vi "VentTrainer.vi"() -> ()   [LabVIEW 2019]
uses:
  <vilib>/Utility/miscctls.llb/LVForegroundBackgroundColorsTypeDef.ctl
  <vilib>/Utility/miscctls.llb/LVTextColorsTypeDef.ctl
  <vilib>/Platform/TimedLoop/XDataNode/timing_clust.ctl
  <vilib>/Platform/TimedLoop/XDataNode/nitl_modes.ctl
  <vilib>/Platform/TimedLoop/XDataNode/wakeup.ctl
  <vilib>/imath/engines/lvmath/Plug In/_Char/NIMS_CH_character datatype.ctl
  <vilib>/numeric/Random Number (Range) U64.vi
  <vilib>/numeric/sub_Random U32.vi
  <vilib>/imath/engines/lvmath2/RunTimeEngine/Managers/WorkSpace/UID Generator.vi
  <vilib>/imath/engines/lvmath2/RunTimeEngine/BuiltInFunctions/le/NIMS_le_no_size_check.vi
  <instcachedir>/0/NIMS_le_no_size_check_D856ED23C6134ED1894787F1ECBE09FB.lvgen/NIMS_le_no_size_check_D856ED23C6134ED1894787F1ECBE09FB_000.vi
  <vilib>/imath/engines/lvmath2/RunTimeEngine/BuiltInFunctions/gt/NIMS_gt_no_size_check.vi
  <instcachedir>/0/NIMS_gt_no_size_check_38A9727757664B91B08F4CCA058B820F.lvgen/NIMS_gt_no_size_check_38A9727757664B91B08F4CCA058B820F_000.vi
  <vilib>/imath/engines/lvmath2/RunTimeEngine/RunTimeType/NIMS_RunTimeType_From StrictType (excl LVString).vi
  <instcachedir>/0/NIMS_RunTimeType_From StrictType (excl LVString)_D8AFBA86A94845AAA577C895450664BD.lvgen/NIMS_RunTimeType_From StrictType (excl LVString)_D8AFBA86A94845AAA577C895450664BD_000.vi
  <vilib>/imath/engines/lvmath2/RunTimeEngine/LocalVariableDefStatement/MC_LocalVariableDefStatement_Display.vi
  <vilib>/imath/engines/lvmath2/RunTimeEngine/Managers/SymbolTable/Clear UID.vi
  <vilib>/imath/engines/lvmath2/RunTimeEngine/NodeEndStatement/NIMS_NodeEndStatement_Output.vi
  <instcachedir>/0/NIMS_NodeEndStatement_Output_53EC0D466D134D7ABD903AC30B43404B.lvgen/NIMS_NodeEndStatement_Output_53EC0D466D134D7ABD903AC30B43404B_001.vi
  <vilib>/imath/engines/lvmath2/RunTimeEngine/ErrorHandling/NIMS_Finalize Error.vi
  <vilib>/imath/engines/lvmath2/RunTimeEngine/BuiltInFunctions/lt/NIMS_lt_no_size_check.vi
  <instcachedir>/0/NIMS_lt_no_size_check_D875779DF14246DBB85DAA0AEACCEBA5.lvgen/NIMS_lt_no_size_check_D875779DF14246DBB85DAA0AEACCEBA5_000.vi
  <vilib>/imath/engines/lvmath/Plug In/_Char/NIMS_CH_Character RV to String.vi
  <instcachedir>/0/NIMS_NodeEndStatement_Output_53EC0D466D134D7ABD903AC30B43404B.lvgen/NIMS_NodeEndStatement_Output_53EC0D466D134D7ABD903AC30B43404B_008.vi
  <instcachedir>/0/NIMS_NodeEndStatement_Output_53EC0D466D134D7ABD903AC30B43404B.lvgen/NIMS_NodeEndStatement_Output_53EC0D466D134D7ABD903AC30B43404B_010.vi
  <vilib>/imath/engines/lvmath2/RunTimeEngine/BuiltInFunctions/ge/NIMS_ge_no_size_check.vi
  <instcachedir>/0/NIMS_ge_no_size_check_103862EFDADA4303A5E7B19FE76B9AA5.lvgen/NIMS_ge_no_size_check_103862EFDADA4303A5E7B19FE76B9AA5_000.vi
  <vilib>/imath/engines/lvmath2/RunTimeEngine/BuiltInFunctions/rem/NIMS_rem_no checks.vi
  <instcachedir>/0/NIMS_rem_no checks_044AAE96F86F43668F02B1B11ED2BED0.lvgen/NIMS_rem_no checks_044AAE96F86F43668F02B1B11ED2BED0_000.vi
  <vilib>/imath/engines/lvmath2/RunTimeSupport/NIMS_Error if Not Equal.vi
  <instcachedir>/0/NIMS_Error if Not Equal_D50A0F08CBFC40E0B64682CCD852CBC7.lvgen/NIMS_Error if Not Equal_D50A0F08CBFC40E0B64682CCD852CBC7_000.vi
  <vilib>/imath/engines/lvmath2/RunTimeEngine/IndexReplace/NIMS V(S)=S.vi
  <instcachedir>/0/NIMS V(S)=S_BD5C8CB81B6E4D99B8C0034EA1BEE55D.lvgen/NIMS V(S)=S_BD5C8CB81B6E4D99B8C0034EA1BEE55D_000.vi
  <vilib>/imath/engines/lvmath2/RunTimeEngine/ErrorHandling/NIMS_Create Error From Enums.vi
  <vilib>/imath/engines/lvmath2/RunTimeEngine/RangeToken/NIMS_Range_R2 - Integer.vi
  <instcachedir>/0/NIMS_Range_R2 - Integer_8A7AF97FD8504F909FC0FDE0F1D1FB54.lvgen/NIMS_Range_R2 - Integer_8A7AF97FD8504F909FC0FDE0F1D1FB54_000.vi
  <vilib>/imath/engines/lvmath2/RunTimeEngine/CommandStatement/MC_CommandStatement_break.vi
  <vilib>/imath/engines/lvmath2/RunTimeEngine/IndexRead/NIMS V(S).vi
  <instcachedir>/0/NIMS V(S)_0488751826AF41519A22953C041130DC.lvgen/NIMS V(S)_0488751826AF41519A22953C041130DC_000.vi
  <vilib>/imathl/engines/lvmath/Functions/Error Handling/Create Error.vi
  <vilib>/imath/engines/lvmath2/RunTimeEngine/VariableToken/NIMS_VariableToken_CondDefined.vi
  <instcachedir>/0/NIMS_VariableToken_CondDefined_30C3C94EAC01413DA882E848DEC89944.lvgen/NIMS_VariableToken_CondDefined_30C3C94EAC01413DA882E848DEC89944_003.vi
  <vilib>/imath/engines/lvmath/Functions/Error Handling/MergeErrorsWrapper.vi
  <instcachedir>/0/NIMS_NodeEndStatement_Output_53EC0D466D134D7ABD903AC30B43404B.lvgen/NIMS_NodeEndStatement_Output_53EC0D466D134D7ABD903AC30B43404B_005.vi
  <instcachedir>/0/NIMS_NodeEndStatement_Output_53EC0D466D134D7ABD903AC30B43404B.lvgen/NIMS_NodeEndStatement_Output_53EC0D466D134D7ABD903AC30B43404B_011.vi
  <instcachedir>/0/NIMS V(S)=S_BD5C8CB81B6E4D99B8C0034EA1BEE55D.lvgen/NIMS V(S)=S_BD5C8CB81B6E4D99B8C0034EA1BEE55D_003.vi
  <vilib>/imath/engines/lvmath2/RunTimeEngine/RangeToken/NIMS_Range_R2 - Float.vi
  <instcachedir>/0/NIMS_Range_R2 - Float_E92E97654E134110B10F16A3994F6405.lvgen/NIMS_Range_R2 - Float_E92E97654E134110B10F16A3994F6405_000.vi
  <vilib>/imath/engines/lvmath2/RunTimeEngine/BuiltInFunctions/eq/NIMS_eq_no_size_check.vi
  <instcachedir>/0/NIMS_eq_no_size_check_3C30971638434A0885768DE8C65273EC.lvgen/NIMS_eq_no_size_check_3C30971638434A0885768DE8C65273EC_000.vi
  <instcachedir>/0/NIMS_NodeEndStatement_Output_53EC0D466D134D7ABD903AC30B43404B.lvgen/NIMS_NodeEndStatement_Output_53EC0D466D134D7ABD903AC30B43404B_012.vi
  <instcachedir>/0/NIMS_NodeEndStatement_Output_53EC0D466D134D7ABD903AC30B43404B.lvgen/NIMS_NodeEndStatement_Output_53EC0D466D134D7ABD903AC30B43404B_018.vi
  <vilib>/platform/TimedLoop/XDataNode/XDataNode.xnode
  <vilib>/Platform/TimedLoop/XDataNode/XDNodeRunTimeDep.lvlib
  <vilib>/imath/engines/lvmath2/RunTimeEngine/Managers/SymbolTable/NIMS_WorkSpace.lvlib
panel:
  out "flagTime1 2":bool
  out "countCycle":dbl
  out "flagTime3":bool
  out "flagTime2":bool
  out "flagTime1":bool
  out "startSimu":bool
  out "indexRef":dbl=1.0
  out "scenTrigger":bool
  out "currentTime":u32=43420372
  out "StringPressure":string="Paw: NaN [cmH2O]\r\nTempo: 0.50 [s]"
  out "StringFlow":string="Fluxo: NaN [l/min]\r\nTempo: 0.50 [s]"
  out "StringVolume":string="Volume: NaN [ml]\r\nTempo: 0.50 [s]"
  out "sizeArray":i32=678
  in  "background":enum32{"Page 1"}(tab)
  in  "info":bool
  out "Bat. %":u8(slide)=100 scale=0.0..100.0
  in  "confTab":enum32{"CONFIGURAÇÕES"}(tab)
  in  "Cenários":u16(ring) items=["Livre", "Cenário 1", "Cenário 2", "Cenário 3", "Cenário 4", "Cenário 5"]
  in  "runBtn":bool
  in  "pacienteTab":T1(tab)
  out "Peso Ideal (kg)":dbl=75.116 format="%_4g"
  in  "Peso (kg)":u16=70 min=1 max=500 step=1
  in  "Altura (m)":dbl=1.8 min=0.1 max=2.8 step=0.1 format="%_2f"
  in  "Idade (anos)":u8=42 min=1 max=120 step=1
  in  "Sexo":u16(ring) items=["Masculino", "Feminino"]
  in  "enbPmus":bool
  in  "enbPalv":bool
  in  "Tempo de Simulação [s]":u8(slide)=10 min=5 max=30 step=5 scale=5.0..30.0
  in  "Rva [cmH2O/l/s]":u8(slide)=10 min=5 max=50 step=2 scale=5.0..50.0
  in  "Cst [ml/cmH2O]":u8(slide)=20 min=5 max=60 step=2 scale=5.0..60.0
  in  "Pausa Inspiratória [s]":dbl(slide) min=0.0 max=5.0 step=0.1 scale=0.0..5.0
  in  "Pmus [cmH2O]":dbl(slide)=2.0999999999999996 min=0.0 max=10.0 step=0.1 scale=0.0..10.0
  in  "stimBtn":bool
  out "spo2":string="SpO2: 97"
  out "alarm_text":string="1  BATERIA fraca"
  in  "ventMode":enum32{"VCV", "PCV"}(tab)
  in  "vcv_blend_up":bool
  in  "vcv_blend_down":bool
  out "vcv_fio2":i16=100
  in  "sens_up":bool
  in  "sens_down":bool
  out "vcv_sens":dbl=-3.0 format="%_2g"
  in  "peep_up":bool
  in  "peep_down":bool
  out "vcv_peep":i16=5
  in  "freq_up":bool
  in  "freq_down":bool
  out "vcv_freq":i16=20
  in  "flow_up":bool
  in  "flow_down":bool
  out "vcv_flow":i16=24
  in  "volume_up":bool
  in  "volume_down":bool
  out "vcv_volume":i16=450
  in  "pc_up":bool
  in  "pc_down":bool
  out "pcv_pc":i16=10
  in  "tinsp_up":bool
  in  "tinsp_down":bool
  out "pcv_tinsp":dbl=1.0 format="%_2g"
  in  "freq_up":bool
  in  "freq_down":bool
  out "pcv_freq":i16=15
  in  "rise_up":bool
  in  "rise_down":bool
  out "pcv_rise":dbl=0.25 format="%.2f"
  in  "peep_up":bool
  in  "peep_down":bool
  out "pcv_peep":i16=5
  in  "sens_up":bool
  in  "sens_down":bool
  out "pcv_sens":dbl=-3.0 format="%_2g"
  in  "blend_up":bool
  in  "blend_down":bool
  out "pcv_blend":i8=100
  in  "monTab":enum32{"MON. 1", "MON. 2"}(tab)
  in  "lowPeak":i16=10 min=0 max=2000 step=1
  in  "highPeak":i16=35 min=0 max=2000 step=1
  out "pPeak":i16
  out "vti":i16
  in  "highVti":i16=400 min=0 max=2000 step=1
  in  "lowVti":i16=200 min=0 max=2000 step=1
  out "ve":dbl format="%.1f"
  in  "highVe":dbl=10.0 min=0.0 max=20.0 step=0.1 format="%_2g"
  in  "lowVe":dbl=2.0 min=0.0 max=20.0 step=0.1 format="%_2f"
  in  "lowPeep":i16=2 min=0 max=2000 step=1
  in  "highPeep":i16=8 min=0 max=2000 step=1
  out "PEEP":dbl format="%_2g"
  in  "lowVte":i16=200 min=0 max=2000 step=1
  in  "highVte":i16=400 min=0 max=2000 step=1
  out "vte":i16
  in  "lowFio2":i16=60 min=21 max=99 step=1
  in  "highFio2":i16=80 min=21 max=100 step=1
  out "Fio2":i16
  out "IE":string="1:0.0"
  out "tInsp":dbl format="%_3g"
  in  "lowFreq":i16=10 min=0 max=2000 step=1
  in  "highFreq":i16=30 min=0 max=2000 step=1
  out "fTotal":i16
  out "pPlateau":dbl
  out "drivingP":dbl
  in  "lowFlow":i16=2 min=0 max=2000 step=1
  in  "highFlow":i16=30 min=0 max=2000 step=1
  out "pFlow":i16
  in  "graphsTab":enum32{"CURVAS", "LOOPs"}(tab)
  out "graph3":cluster{dbl[], dbl[]}[](graph)=[{array[678 elements], array[679 elements]}, {array[678 elements], array[703 elements]}, {array[678 elements], [nan, nan, nan, nan, nan, nan, nan, nan, nan, nan, nan, nan, nan, nan, nan, nan, nan, nan, nan, nan, nan, nan, nan, nan, nan, nan, nan, nan, nan, nan, nan, nan, nan, nan, nan, nan, nan, nan, nan, nan, nan, nan, nan, nan, nan, nan, nan, nan, nan, nan, nan, nan, nan, nan, nan, nan, nan, nan, nan, nan, nan, nan, nan, nan, nan, nan, nan, nan, nan, nan, nan, nan, nan, nan, nan, nan, nan, nan, nan, nan, nan, nan, nan, nan, nan, nan, nan, nan, nan, nan, nan, nan, nan, nan, nan, nan, nan, nan, nan, nan, nan, nan, nan, nan, nan, nan, nan, nan, nan, nan, nan, nan, nan, nan, nan, nan, nan, nan, nan, nan, nan, nan, nan, nan, nan, nan, nan, nan, nan, nan, nan, nan, nan, nan, nan, nan, nan, nan, nan, nan, nan, nan, nan, nan, nan, nan, nan, nan, nan, nan, nan, nan, nan, nan, nan, nan, nan, nan, nan, nan, nan, nan, nan, nan, nan, nan, nan, nan, nan, nan, nan, nan, nan, nan, nan, nan, nan, nan, nan, nan, nan, nan, nan, nan, nan, nan, nan, nan, nan, nan, nan, nan, nan, nan, nan, nan, nan, nan, nan, nan, nan, nan, nan, nan, nan, nan, nan, nan, nan, nan, nan, nan, nan, nan, nan, nan, nan, nan, nan, nan, nan, nan, nan, nan, nan, nan, nan, nan, nan, nan, nan, nan, nan, nan, nan, nan, nan, nan, nan, nan, nan, nan, nan, nan, nan, nan, nan, nan, nan, nan, nan, nan, nan, nan, nan, nan, nan, nan, nan, nan, nan, nan, nan, nan, nan, nan, nan, nan, nan, nan, nan, nan, nan, nan, nan, nan, nan, nan, nan, nan, nan, nan, nan, nan, nan, nan, nan, nan, nan, nan, nan, nan, nan, nan, nan, nan, nan, nan, nan, nan, nan, nan, nan, nan, nan, nan, nan, nan, nan, nan, nan, nan, nan, nan, nan, nan, nan, nan, nan, nan, nan, nan, nan, nan, nan, nan, nan, nan, nan, nan, nan, nan, nan, nan, nan, nan, nan, nan, nan, nan, nan, nan, nan, nan, nan, nan, nan, nan, nan, nan, nan, nan, nan, nan, nan, nan, nan, nan, nan, nan, nan, nan, nan, nan, nan, nan, nan, nan, nan, nan, nan, nan, nan, nan, nan, nan, nan, nan, nan, nan, nan, nan, nan, nan, nan, nan, nan, nan, nan, nan, nan, nan, nan, nan, nan, nan, nan, nan, nan, nan, nan, nan, nan, nan, nan, nan, nan, nan, nan, nan, nan, nan, nan, nan, nan, nan, nan, nan, nan, nan, nan, nan, nan, nan, nan, nan, nan, nan, nan, nan, nan, nan, nan, nan, nan, nan, nan, nan, nan, nan, nan, nan, nan, nan, nan, nan, nan, nan, nan, nan, nan, nan, nan, nan, nan, nan, nan, nan, nan, nan, nan, nan, nan, nan, nan, nan, nan, nan, nan, nan, nan, nan, nan, nan, nan, nan, nan, nan, nan, nan, nan, nan, nan, nan, nan, nan, nan, nan, nan, nan, nan, nan, nan, nan, nan, nan, nan, nan, nan, nan, nan, nan, nan, nan, nan, nan, nan, nan, nan, nan, nan, nan, nan, nan, nan, nan, nan, nan, nan, nan, nan, nan, nan, nan, nan, nan, nan, nan, nan, nan, nan, nan, nan, nan, nan, nan, nan, nan, nan, nan, nan, nan, nan, nan, nan, nan, nan, nan, nan, nan, nan, nan, nan, nan, nan, nan, nan, nan, nan, nan, nan, nan, nan, nan, nan, nan, nan, nan, nan, nan, nan, nan, nan, nan, nan, nan, nan, nan, nan, nan, nan, nan, nan, nan, nan, nan, nan, nan, nan, nan, nan, nan, nan, nan, nan, nan, nan, nan, nan, nan, nan, nan, nan, nan, nan, nan, nan, nan, nan, nan, nan, nan, nan, nan, nan, nan, nan, nan, nan, nan, nan, nan, nan, nan, nan, nan, nan, nan, nan, nan, nan, nan, nan, nan, nan, nan, nan, nan, nan, nan, nan, nan, nan, nan, nan, nan, nan, nan, nan, nan, nan, nan, nan, nan, nan, nan, nan, nan, nan, nan, nan, nan, nan, nan, nan, nan, nan, nan, nan, nan, nan, nan, nan, nan, nan, nan, nan, nan, nan, nan, nan, nan, nan, nan, nan, nan, nan, nan, nan, nan, nan, nan, nan, nan, nan, nan, nan, nan, nan, nan, nan, nan, nan]}, {array[678 elements], [nan, nan, nan, nan, nan, nan, nan, nan, nan, nan, nan, nan, nan, nan, nan, nan, nan, nan, nan, nan, nan, nan, nan, nan, nan, nan, nan, nan, nan, nan, nan, nan, nan, nan, nan, nan, nan, nan, nan, nan, nan, nan, nan, nan, nan, nan, nan, nan, nan, nan, nan, nan, nan, nan, nan, nan, nan, nan, nan, nan, nan, nan, nan, nan, nan, nan, nan, nan, nan, nan, nan, nan, nan, nan, nan, nan, nan, nan, nan, nan, nan, nan, nan, nan, nan, nan, nan, nan, nan, nan, nan, nan, nan, nan, nan, nan, nan, nan, nan, nan, nan, nan, nan, nan, nan, nan, nan, nan, nan, nan, nan, nan, nan, nan, nan, nan, nan, nan, nan, nan, nan, nan, nan, nan, nan, nan, nan, nan, nan, nan, nan, nan, nan, nan, nan, nan, nan, nan, nan, nan, nan, nan, nan, nan, nan, nan, nan, nan, nan, nan, nan, nan, nan, nan, nan, nan, nan, nan, nan, nan, nan, nan, nan, nan, nan, nan, nan, nan, nan, nan, nan, nan, nan, nan, nan, nan, nan, nan, nan, nan, nan, nan, nan, nan, nan, nan, nan, nan, nan, nan, nan, nan, nan, nan, nan, nan, nan, nan, nan, nan, nan, nan, nan, nan, nan, nan, nan, nan, nan, nan, nan, nan, nan, nan, nan, nan, nan, nan, nan, nan, nan, nan, nan, nan, nan, nan, nan, nan, nan, nan, nan, nan, nan, nan, nan, nan, nan, nan, nan, nan, nan, nan, nan, nan, nan, nan, nan, nan, nan, nan, nan, nan, nan, nan, nan, nan, nan, nan, nan, nan, nan, nan, nan, nan, nan, nan, nan, nan, nan, nan, nan, nan, nan, nan, nan, nan, nan, nan, nan, nan, nan, nan, nan, nan, nan, nan, nan, nan, nan, nan, nan, nan, nan, nan, nan, nan, nan, nan, nan, nan, nan, nan, nan, nan, nan, nan, nan, nan, nan, nan, nan, nan, nan, nan, nan, nan, nan, nan, nan, nan, nan, nan, nan, nan, nan, nan, nan, nan, nan, nan, nan, nan, nan, nan, nan, nan, nan, nan, nan, nan, nan, nan, nan, nan, nan, nan, nan, nan, nan, nan, nan, nan, nan, nan, nan, nan, nan, nan, nan, nan, nan, nan, nan, nan, nan, nan, nan, nan, nan, nan, nan, nan, nan, nan, nan, nan, nan, nan, nan, nan, nan, nan, nan, nan, nan, nan, nan, nan, nan, nan, nan, nan, nan, nan, nan, nan, nan, nan, nan, nan, nan, nan, nan, nan, nan, nan, nan, nan, nan, nan, nan, nan, nan, nan, nan, nan, nan, nan, nan, nan, nan, nan, nan, nan, nan, nan, nan, nan, nan, nan, nan, nan, nan, nan, nan, nan, nan, nan, nan, nan, nan, nan, nan, nan, nan, nan, nan, nan, nan, nan, nan, nan, nan, nan, nan, nan, nan, nan, nan, nan, nan, nan, nan, nan, nan, nan, nan, nan, nan, nan, nan, nan, nan, nan, nan, nan, nan, nan, nan, nan, nan, nan, nan, nan, nan, nan, nan, nan, nan, nan, nan, nan, nan, nan, nan, nan, nan, nan, nan, nan, nan, nan, nan, nan, nan, nan, nan, nan, nan, nan, nan, nan, nan, nan, nan, nan, nan, nan, nan, nan, nan, nan, nan, nan, nan, nan, nan, nan, nan, nan, nan, nan, nan, nan, nan, nan, nan, nan, nan, nan, nan, nan, nan, nan, nan, nan, nan, nan, nan, nan, nan, nan, nan, nan, nan, nan, nan, nan, nan, nan, nan, nan, nan, nan, nan, nan, nan, nan, nan, nan, nan, nan, nan, nan, nan, nan, nan, nan, nan, nan, nan, nan, nan, nan, nan, nan, nan, nan, nan, nan, nan, nan, nan, nan, nan, nan, nan, nan, nan, nan, nan, nan, nan, nan, nan, nan, nan, nan, nan, nan, nan, nan, nan, nan, nan, nan, nan, nan, nan, nan, nan, nan, nan, nan, nan, nan, nan, nan, nan, nan, nan, nan, nan, nan, nan, nan, nan, nan, nan, nan, nan, nan, nan, nan, nan, nan, nan, nan, nan, nan, nan, nan, nan, nan, nan, nan, nan, nan, nan, nan, nan, nan, nan, nan, nan, nan, nan, nan, nan, nan, nan, nan, nan, nan, nan, nan, nan, nan, nan, nan, nan, nan, nan, nan, nan, nan, nan, nan, nan, nan, nan, nan, nan, nan, nan, nan, nan, nan, nan, nan, nan, nan, nan]}]
  out "graph1":cluster{"vec_1":dbl[], "vec_2":dbl[]}[](graph)
  out "graph2":cluster{"vec_1":dbl[], "vec_3":dbl[]}[](graph)
  out "graph4":cluster{"vec_2":dbl[], "vec_4":dbl[]}(graph)
  out "graph5":cluster{"vec_2":dbl[], "vec_4":dbl[]}(graph)
  out "trigger":bool
  out "rstModel":bool
  out "flag1":bool
  out "timeRef1":dbl=0.5
  out "flag3":bool
  out "timeRef3":dbl=8.040000000000001
  out "flag2":bool
  out "timeRef2":dbl=6.96 format="%.2f"
  out "scaleTrigger":bool
  out "simuTime":u8=10
  out "minFlow":dbl=-98.76291251592673
  out "maxFlow":dbl=24.0
  out "initTime":u64=43388394
  out "graphPressure":dbl format="%.6f"
  # "FiO2"
  # "%"
  # "Sens"
  # "cmH2O"
  # "PEEP"
  # "cmH2O"
  # "Freq"
  # "rpm"
  # "Flow"
  # "L/min"
  # "Volume"
  # "ml"
  # "PC"
  # "cmH2O"
  # "T. Insp"
  # "s"
  # "Freq"
  # "rpm"
  # "Rise Time"
  # "s"
  # "PEEP"
  # "cmH2O"
  # "Sens"
  # "cmH2O"
  # "FiO2"
  # "%"
  # "P. Peak"
  # "cmH2O"
  # "VTI"
  # "ml"
  # "VE"
  # "L/min"
  # "PEEP"
  # "cmH2O"
  # "VTE"
  # "ml"
  # "FiO2"
  # "%"
  # "I:E"
  # "T. Insp"
  # "s"
  # "fTotal"
  # "rpm"
  # "P. Plateau"
  # "cmH2O"
  # "Driving P."
  # "cmH2O"
  # "Peak Flow"
  # "ml/min"
  # "Volume [ml]"
  # "Fluxo [l/min]"
  # "Pressão [cmH2O]"
  # "Tempo [s]"
  # "Volume [ml]"
  # "Pressão [cmH2O]"
  # "Fluxo [L/min]"
  # "Volume [ml]"
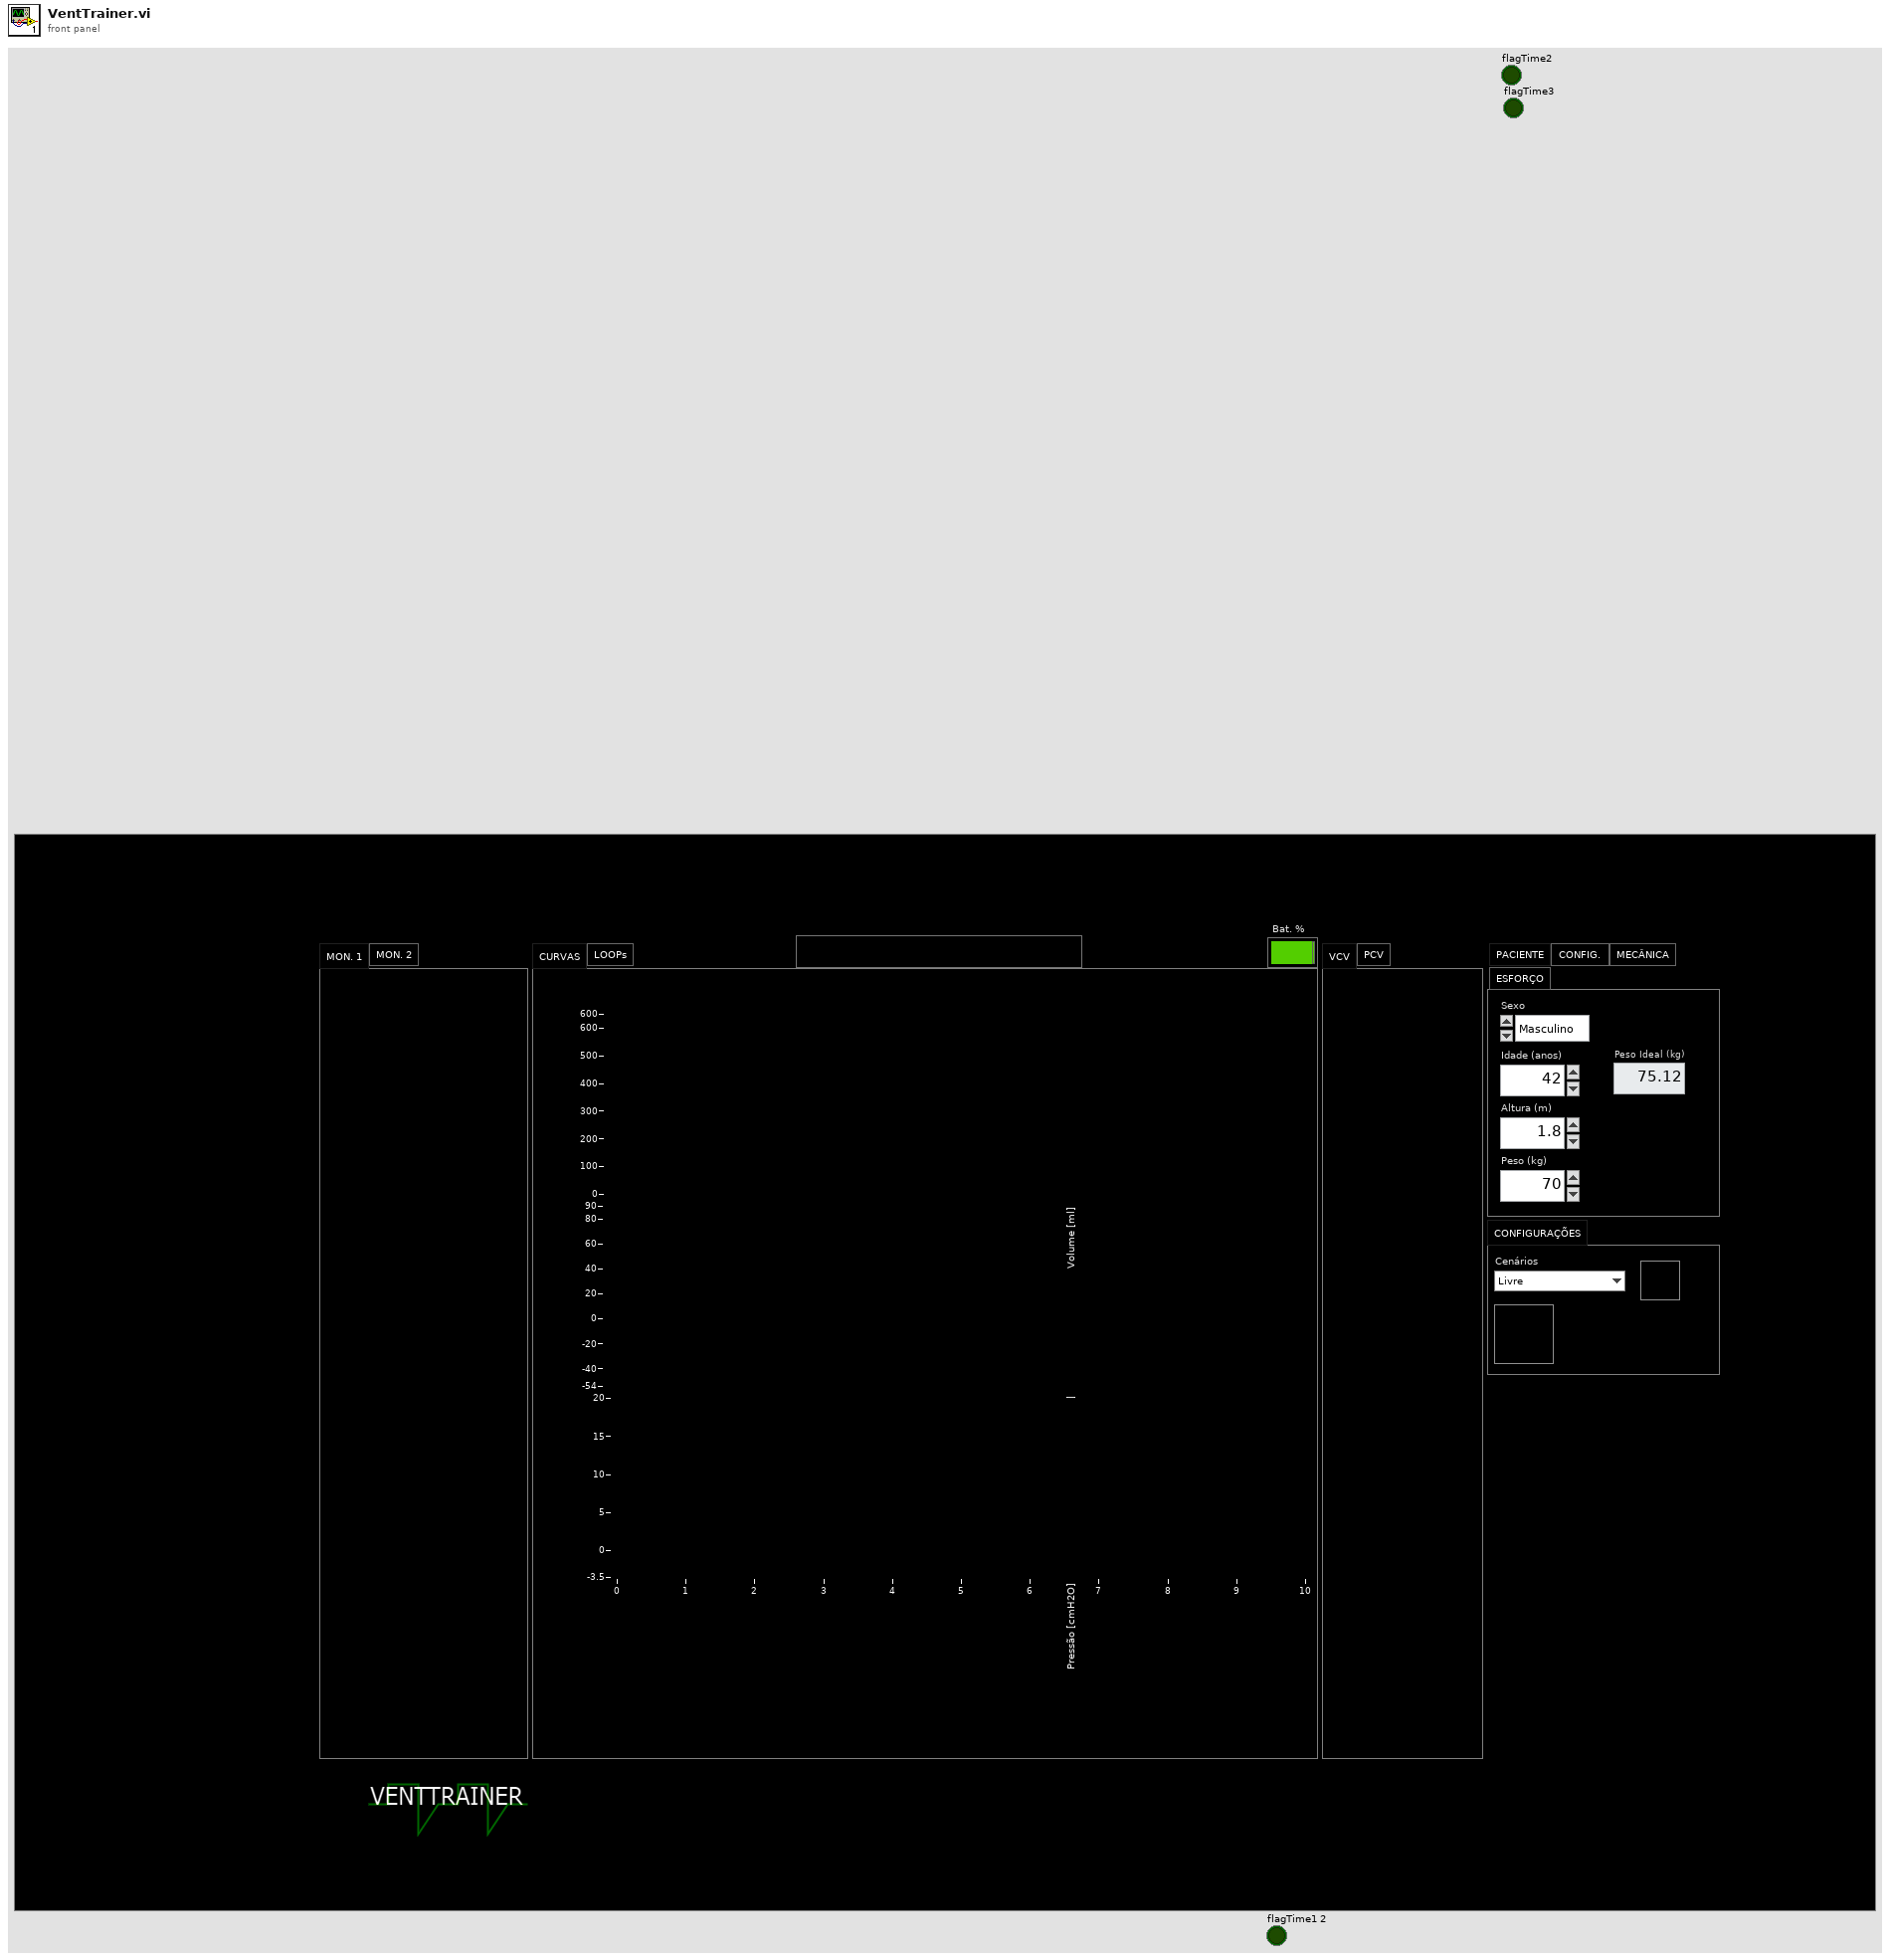
[diagram p1: front panel]
types:
  T1 = enum32{"PACIENTE", "CONFIG. ", "MECÂNICA", "ESFORÇO"}
  T2 = typedef "LVTextColorsTypeDef.ctl" = cluster{"Text Color":u32, "Background Color":u32}
  T3 = typedef "LVForegroundBackgroundColorsTypeDef.ctl" = cluster{"Foreground Color":u32, "Background Color":u32}
  T4 = typedef "XDNodeRunTimeDep.lvlib/timing_clust.ctl" = cluster{"Expected End [f-1]":u64, "Actual End [f-1]":u64, "Finished Late? [f-1]":bool, "Expected End [i-1]":u64, "Actual End [i-1]":u64, "Finished Late? [i-1]":bool, "Expected Start [i]":u64, "Actual Start [i]":u64, "Expected Start [f]":u64, "Actual Start [f]":u64, "Source Name":string, "Structure Name":string, "Period":i64, "Deadline":i64, "Offset":i64, "Start":i64, "Priority":i32, "Timeout":i32, "Mode":T5, "Wakeup Reason":T6, "Error":errorcluster, "Source Type":string, "Secondary Source Type":string, "Global End Time":u64, "Global Start Time":u64, "Frame Duration":u64, "Iteration Duration":u64, "Assigned CPU":i32, "I/O Scan Engine Mode":u32}
  T5 = typedef "XDNodeRunTimeDep.lvlib/nitl_modes.ctl" = enum32{"No Change", "Process missed periods, maintain original phase", "Discard missed periods, maintain original phase", "Process missed periods, ignore original phase", "Discard missed periods, ignore original phase"}
  T6 = typedef "XDNodeRunTimeDep.lvlib/wakeup.ctl" = enum32{"Normal", "Aborted", "Asynchronous wakeup", "Timing source error", "Timed loop error", "Timeout"}
  T7 = enum8{"Enabled", "Disabled", "Disabled and Grayed Out"}
  T8 = typedef "NIMS_CH_character datatype.ctl" = cluster{"Numeric":u8}
  T9 = typedef "LVPoint32TypeDef.ctl" = cluster{"Horizontal":i32, "Vertical":i32}
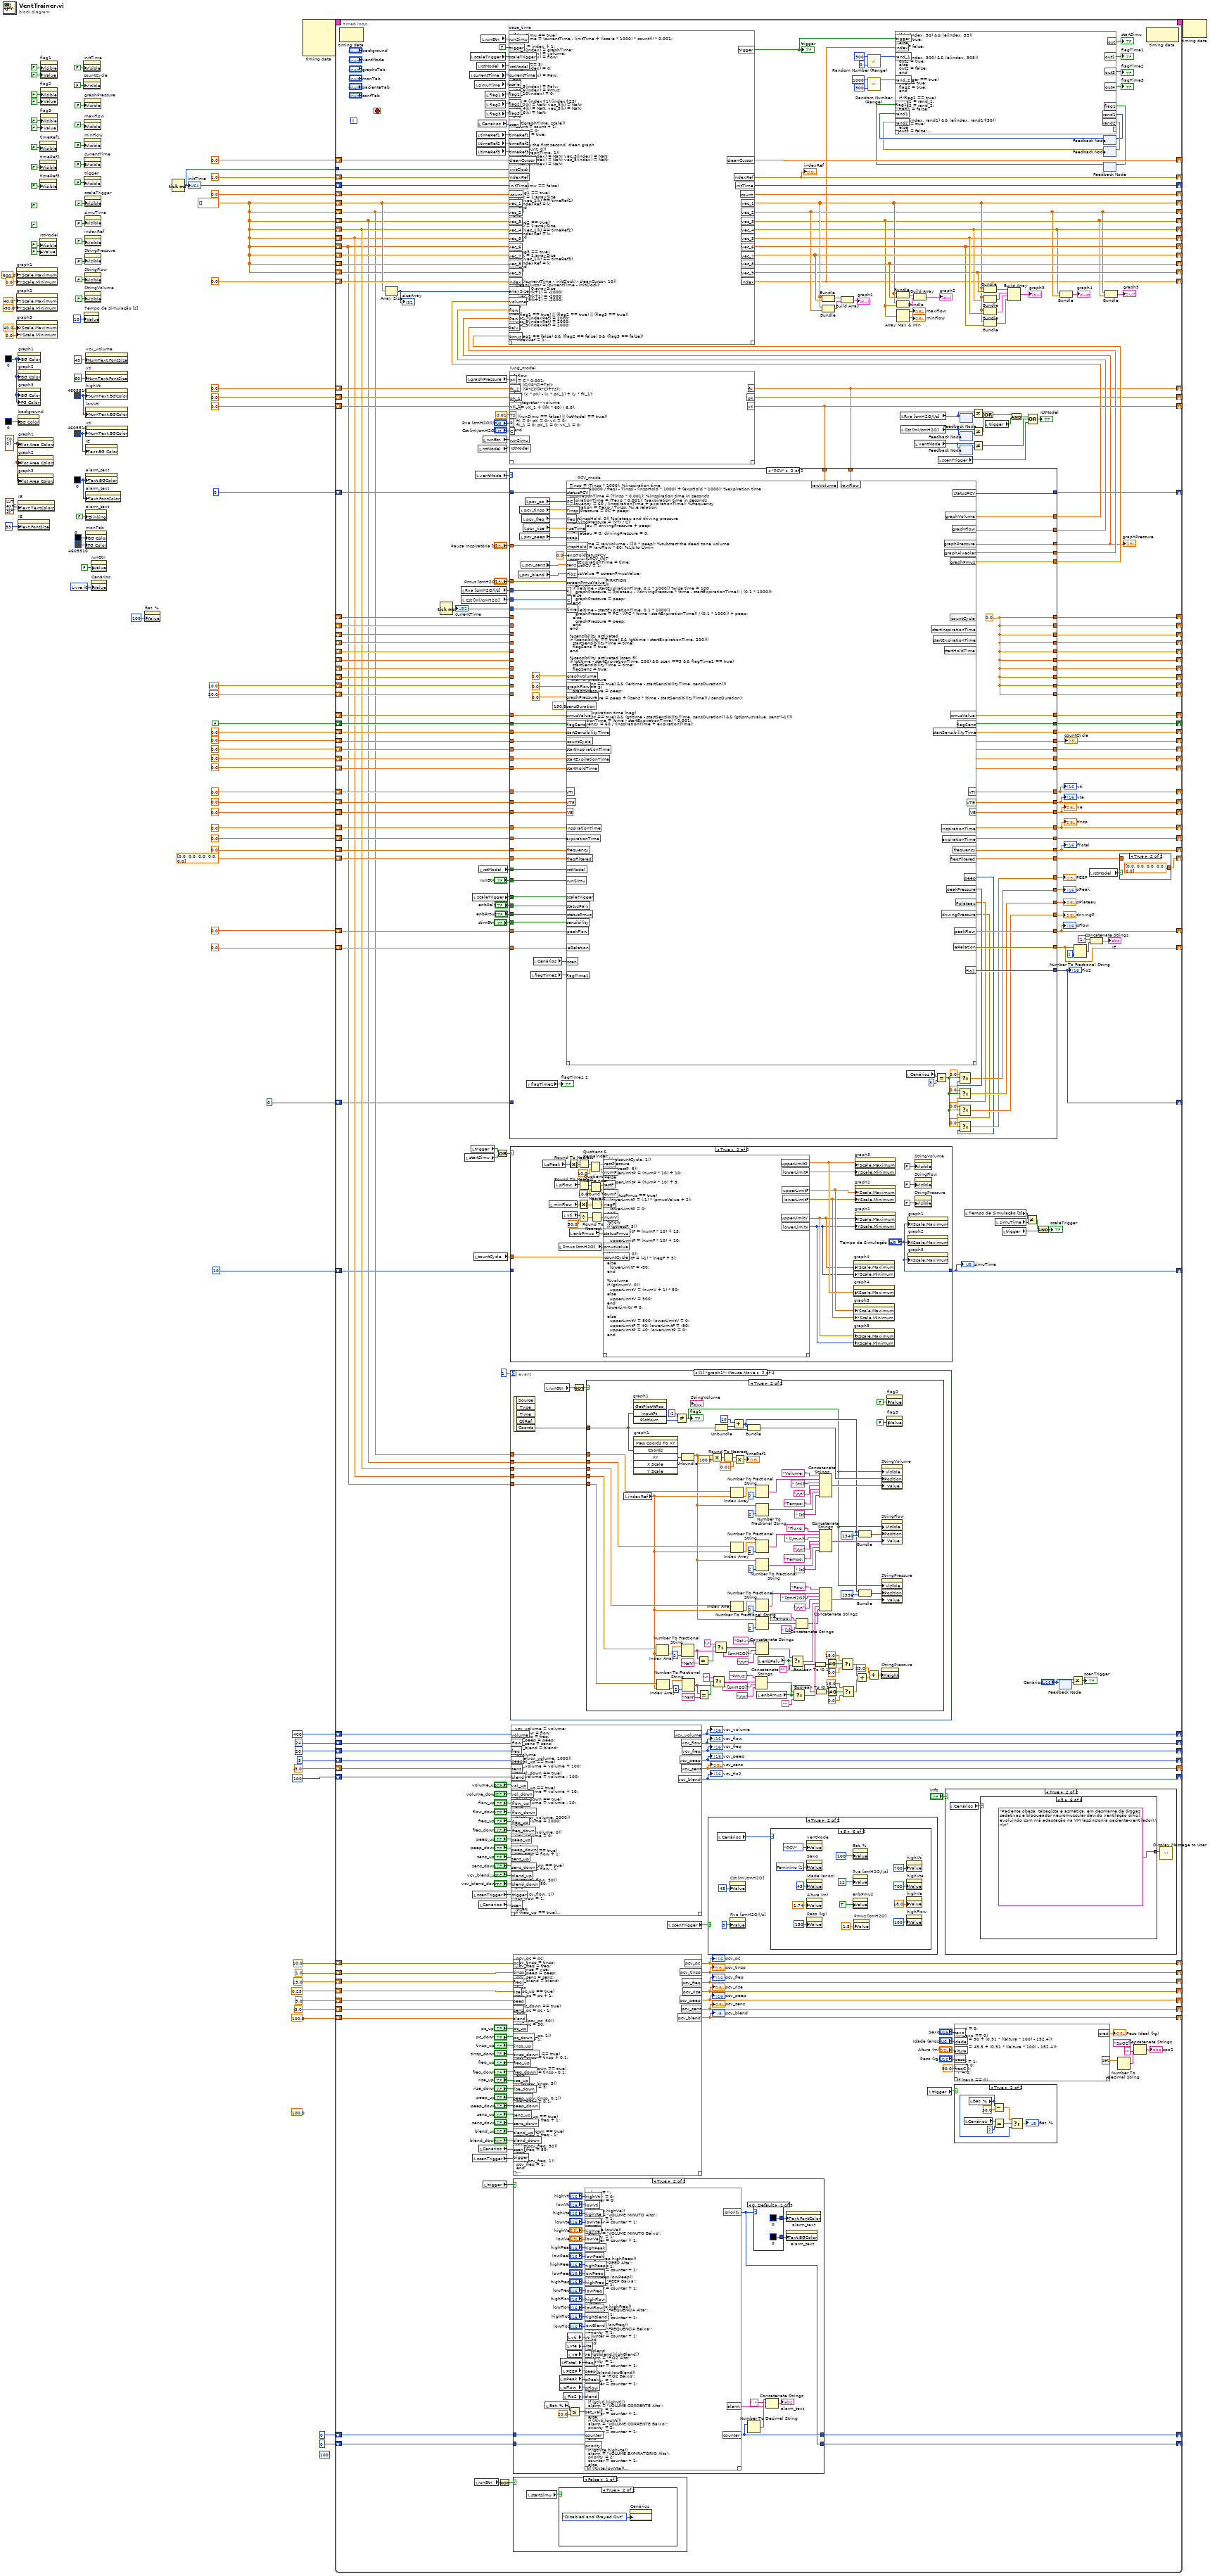
[diagram p0: block diagram]
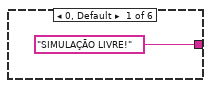
[diagram p4: hidden frame]
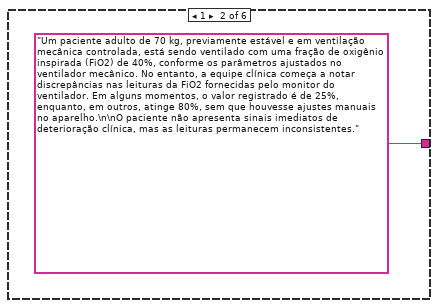
[diagram p5: hidden frame]
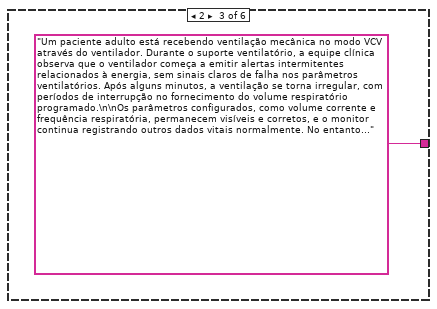
[diagram p6: hidden frame]
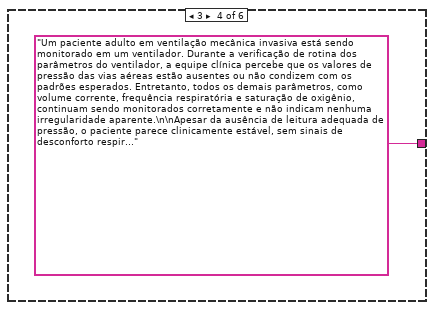
[diagram p7: hidden frame]
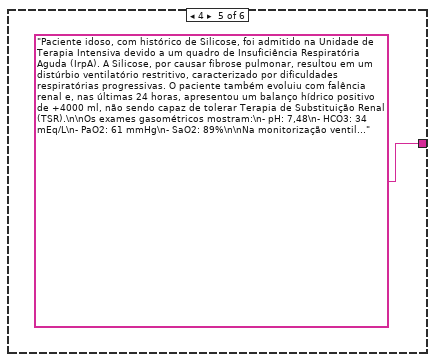
[diagram p8: hidden frame]
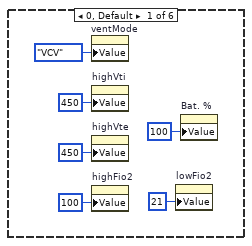
[diagram p11: hidden frame]
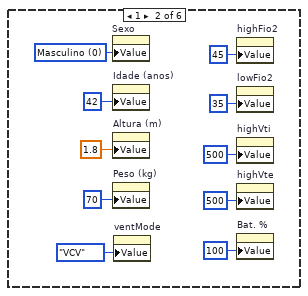
[diagram p12: hidden frame]
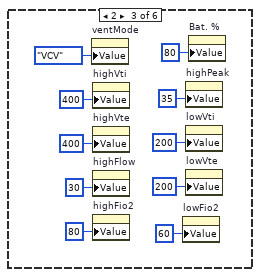
[diagram p13: hidden frame]
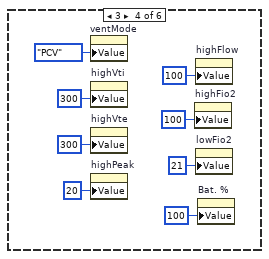
[diagram p14: hidden frame]
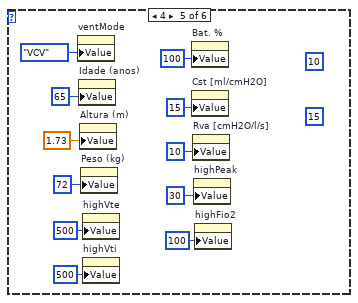
[diagram p15: hidden frame]
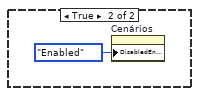
[diagram p17: hidden frame]
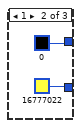
[diagram p19: hidden frame]
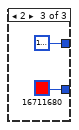
[diagram p20: hidden frame]
diagram:
  (unwired) 100
  (unwired) 100.0 ("x")
  w4 = u16 0 items=["Livre", "Técnico 1", "Técnico 2", "Técnico 3", "Operacional 1", "Operacional 2"] ("Cenários")
  w14 = u32 0 ("Colors:BG Color")
  w29 = u32 4605510 ("Plot Area:Colors:BG Color")
  w31 = u32 4605510 ("Text.Text Colors:BG Color")
  w33 = T3 {"Foreground Color"=0, "Background Color"=0} ("Plot Area:Colors")
  w30 = u32 0 ("Plot Area:Colors:BG Color")
  (unwired) FALSE
  (unwired) FALSE
  w45 = dbl[] [] ("vec_1")
  n1 = property on="graph1" class="XYGraph (strict)"("YScale.Maximum"=500.0 ("Y Scale.Range:Maximum"), "YScale.Minimum"=0.0 ("Y Scale.Range:Minimum")) -> ()  [unwired: 2 in, 2 out]
  n2 = property on="graph2" class="XYGraph (strict)"("YScale.Maximum"=40.0 ("Y Scale.Range:Maximum"), "YScale.Minimum"=-90.0 ("Y Scale.Range:Minimum")) -> ()  [unwired: 2 in, 2 out]
  n3 = property on="graph3" class="XYGraph (strict)"("YScale.Maximum"=40.0 ("Y Scale.Range:Maximum"), "YScale.Minimum"=0.0 ("Y Scale.Range:Minimum")) -> ()  [unwired: 2 in, 2 out]
  n4 = property on="graph1" class="XYGraph (strict)"("BG Color"=w30) -> ()  [unwired: 2 in, 2 out]
  n5 = property on="graph2" class="XYGraph (strict)"("BG Color"=w30) -> ()  [unwired: 2 in, 2 out]
  n6 = property on="graph3" class="XYGraph (strict)"("BG Color"=w30, "FG Color"=w30) -> ()  [unwired: 2 in, 2 out]
  n7 = property on="background" class="TabCtl (strict)"("BG Color"=u32 0 ("Plot Area:Colors:BG Color")) -> ()  [unwired: 2 in, 2 out]
  n8 = property on="graph1" class="XYGraph (strict)"("Plot Area Colors"=w33) -> ()  [unwired: 2 in, 2 out]
  n9 = property on="graph2" class="XYGraph (strict)"("Plot Area Colors"=w33) -> ()  [unwired: 2 in, 2 out]
  n10 = property on="graph3" class="XYGraph (strict)"("Plot Area Colors"=w33) -> ()  [unwired: 2 in, 2 out]
  n11 = property on="IE" class="Str"("Text.TextColors"=T2 {"Text Color"=16777225, "Background Color"=4605510} ("Text.Text Colors")) -> ()  [unwired: 2 in, 2 out]
  n12 = property on="IE" class="Str"("Text.FontSize"=u32 55 ("Text.Font:Size")) -> ()  [unwired: 2 in, 2 out]
  n13 = property on="timeRef1" class="DigNum (strict)"("Visible"=FALSE) -> ()  [unwired: 2 in, 2 out]
  n14 = property on="timeRef2" class="DigNum (strict)"("Visible"=FALSE) -> ()  [unwired: 2 in, 2 out]
  n15 = property on="timeRef3" class="DigNum (strict)"("Visible"=FALSE) -> ()  [unwired: 2 in, 2 out]
  n16 = property on="rstModel" class="Bool (strict)"("Visible"=FALSE, "Value"=FALSE) -> ()  [unwired: 2 in, 2 out]
  n17 = property on="flag1" class="Bool (strict)"("Visible"=FALSE, "Value"=FALSE) -> ()  [unwired: 2 in, 2 out]
  n18 = property on="flag2" class="Bool (strict)"("Visible"=FALSE, "Value"=FALSE) -> ()  [unwired: 2 in, 2 out]
  n19 = property on="flag3" class="Bool (strict)"("Visible"=FALSE, "Value"=FALSE) -> ()  [unwired: 2 in, 2 out]
  n20 = property on="initTime" class="DigNum (strict)"("Visible"=FALSE) -> ()  [unwired: 2 in, 2 out]
  n21 = property on="countCycle" class="DigNum (strict)"("Visible"=FALSE) -> ()  [unwired: 2 in, 2 out]
  n22 = property on="graphPressure" class="DigNum (strict)"("Visible"=FALSE) -> ()  [unwired: 2 in, 2 out]
  n23 = property on="maxFlow" class="DigNum (strict)"("Visible"=FALSE) -> ()  [unwired: 2 in, 2 out]
  n24 = property on="minFlow" class="DigNum (strict)"("Visible"=FALSE) -> ()  [unwired: 2 in, 2 out]
  n25 = property on="currentTime" class="DigNum (strict)"("Visible"=FALSE) -> ()  [unwired: 2 in, 2 out]
  n26 = property on="trigger" class="Bool (strict)"("Visible"=FALSE) -> ()  [unwired: 2 in, 2 out]
  n27 = property on="Tempo de Simulação [s]" class="Slide (strict)"("Value"=u8 10 ("Tempo de simulação [s]")) -> ()  [unwired: 2 in, 2 out]
  n28 = property on="scaleTrigger" class="Bool (strict)"("Visible"=FALSE) -> ()  [unwired: 2 in, 2 out]
  n29 = property on="simuTime" class="DigNum (strict)"("Visible"=FALSE) -> ()  [unwired: 2 in, 2 out]
  n30 = property on="indexRef" class="DigNum (strict)"("Visible"=FALSE) -> ()  [unwired: 2 in, 2 out]
  n31 = property on="StringPressure" class="Str"("Visible"=FALSE) -> ()  [unwired: 2 in, 2 out]
  n32 = property on="StringFlow" class="Str"("Visible"=FALSE) -> ()  [unwired: 2 in, 2 out]
  n33 = property on="StringVolume" class="Str"("Visible"=FALSE) -> ()  [unwired: 2 in, 2 out]
  n34 = property on="vcv_volume" class="DigNum (strict)"("NumText.FontSize"=u32 45 ("Numeric Text.Font:Size")) -> ()  [unwired: 2 in, 2 out]
  n35 = property on="vti" class="DigNum (strict)"("NumText.FontSize"=u32 60 ("Numeric Text.Font:Size")) -> ()  [unwired: 2 in, 2 out]
  n36 = property on="highVti" class="DigNum (strict)"("NumText.BGColor"=w31) -> ()  [unwired: 2 in, 2 out]
  n37 = property on="lowVti" class="DigNum (strict)"("NumText.BGColor"=w31) -> ()  [unwired: 2 in, 2 out]
  n38 = property on="vti" class="DigNum (strict)"("NumText.BGColor"=w29) -> ()  [unwired: 2 in, 2 out]
  n39 = property on="IE" class="Str"("Text.BG Color"=w29) -> ()  [unwired: 2 in, 2 out]
  n40 = property on="alarm_text" class="Str"("Text.BGColor"=w14) -> ()  [unwired: 2 in, 2 out]
  n41 = property on="alarm_text" class="Str"("Text.FontColor"=w14) -> ()  [unwired: 2 in, 2 out]
  n42 = property on="alarm_text" class="Str"("Blinking"=FALSE) -> ()  [unwired: 2 in, 2 out]
  n43 = property on="monTab" class="TabCtl (strict)"("BG Color"=u32 0 ("Colors:BG Color"), "FG Color"=u32 4605510 ("Colors:BG Color")) -> ()  [unwired: 2 in, 2 out]
  n44 = property on="runBtn" class="Bool (strict)"("Value"=FALSE ("runBtn")) -> ()  [unwired: 2 in, 2 out]
  n45 = property on="Cenários" class="Ring (strict)"("Value"=w4) -> ()  [unwired: 2 in, 2 out]
  n46 = property on="Bat. %" class="Slide (strict)"("Value"=u8 100 ("Bat. %")) -> ()  [unwired: 2 in, 2 out]
  n47 = Tick Count (ms)() -> (millisecond timer value=w43:u32)
  "initTime" <- w43
  n48 = node-c288() -> (w93:T4)  [unwired: 4 in]
  n49 = timed-loop {
    timing: w93 -> [_]
    timing-out: [_] -> w92
    shift-right: [w317] -> _
    shift-left: 0.0 ("uK") -> [w316]
    shift-right: [w248] -> _
    shift-left: 0.0 ("yK") -> [w362]
    shift-right: [w345] -> _
    shift-left: 0 -> [w263]
    shift-right: [w364] -> _
    shift-left: 0.0 ("startExpirationTime") -> [w367]
    shift-right: [w363] -> _
    shift-left: 0.0 ("startInspirationTime") -> [w368]
    shift-right: [w365] -> _
    shift-left: 0.0 ("startExpirationTime") -> [w366]
    shift-right: [w353] -> _
    shift-left: 0.0 ("xK") -> [w361]
    shift-right: [w153] -> _
    shift-left: 0.0 ("VTI") -> [w360]
    shift-right: [w152] -> _
    shift-left: 0.0 ("VTE") -> [w359]
    shift-right: [w151] -> _
    shift-left: 0.0 ("VE") -> [w358]
    shift-right: [w246] -> _
    shift-left: 0.0 ("VE") -> [w354]
    shift-right: [w351] -> _
    shift-left: 0.0 ("count") -> [w352]
    shift-right: [w350] -> _
    shift-left: w43 -> [w348]
    shift-right: [w347] -> _
    shift-left: 0.0 ("countCycle") -> [w346]
    shift-right: [w338] -> _
    shift-left: 0.0 ("sensTime") -> [w337]
    shift-right: [w335] -> _
    shift-left: FALSE -> [w336]
    shift-right: [w150] -> _
    shift-left: 0.0 ("VE") -> [w334]
    shift-right: [w332] -> _
    shift-left: 0.0 ("VE") -> [w333]
    shift-right: [w149] -> _
    shift-left: 0.0 ("VE") -> [w331]
    shift-right: [w330] -> _
    shift-left: 0.0 ("VE") -> [w329]
    shift-right: [w173] -> _
    shift-left: w45 -> [w302]
    shift-right: [w168] -> _
    shift-left: w45 -> [w175]
    shift-right: [w170] -> _
    shift-left: w45 -> [w179]
    shift-right: [w169] -> _
    shift-left: w45 -> [w178]
    shift-right: [w322] -> _
    shift-left: w45 -> [w176]
    shift-right: [w236] -> _
    shift-left: w45 -> [w177]
    shift-right: [w120] -> _
    shift-left: 0.0 ("index") -> [w323]
    shift-right: [w208] -> _
    shift-left: u8 10 ("Tempo de simulação [s]") -> [w311]
    shift-right: [w288] -> _
    shift-left: 1.0 ("indexRef") -> [w299]
    shift-right: [w289] -> _
    shift-left: w45 -> [w298]
    shift-right: [w284] -> _
    shift-left: w45 -> [w297]
    shift-right: [w282] -> _
    shift-left: w45 -> [w296]
    shift-right: [w292] -> _
    shift-left: 0.0 ("clean") -> [w291]
    tunnel: w43 -> [w290]
    shift-right: [w280] -> _
    shift-left: _ -> [w281]
    shift-right: [w279] -> _
    shift-left: _ -> [w271]
    shift-right: [w278] -> _
    shift-left: _ -> [w270]
    shift-right: [w277] -> _
    shift-left: _ -> [w269]
    shift-right: [w276] -> _
    shift-left: _ -> [w268]
    shift-right: [w275] -> _
    shift-left: _ -> [w267]
    shift-right: [w274] -> _
    shift-left: _ -> [w266]
    shift-right: [w273] -> _
    shift-left: _ -> [w265]
    shift-right: [w272] -> _
    shift-left: _ -> [w264]
    shift-right: [w125] -> _
    shift-left: dbl[] [0.0, 0.0, 0.0, 0.0, 0.0] ("freqFiltered") -> [w258]
    shift-right: [w257] -> _
    shift-left: 10.0 ("R") -> [w255]
    shift-right: [w256] -> _
    shift-left: 20.0 ("C") -> [w254]
    shift-right: [w214] -> _
    shift-left: 400 ("vcv_volume") -> [w232]
    shift-right: [w213] -> _
    shift-left: 24 ("vcv_flow") -> [w231]
    shift-right: [w210] -> _
    shift-left: 20 ("vcv_freq") -> [w230]
    shift-right: [w211] -> _
    shift-left: 5 ("vcv_peep") -> [w229]
    shift-right: [w212] -> _
    shift-left: -3.0 ("vcv_sens") -> [w228]
    shift-right: [w136] -> _
    shift-left: 100 ("vcv_blend") -> [w227]
    shift-right: [w180] -> _
    shift-left: 10.0 ("x") -> [w207]
    shift-right: [w181] -> _
    shift-left: 1.0 ("x") -> [w206]
    shift-right: [w182] -> _
    shift-left: 15.0 ("x") -> [w205]
    shift-right: [w183] -> _
    shift-left: 0.25 ("x") -> [w204]
    shift-right: [w184] -> _
    shift-left: 5.0 ("x") -> [w203]
    shift-right: [w185] -> _
    shift-left: -3.0 ("x") -> [w202]
    shift-right: [w186] -> _
    shift-left: 100.0 ("x") -> [w201]
    shift-right: [w165] -> _
    shift-left: 0 -> [w166]
    shift-right: [w96] -> _
    shift-left: u64 0 ("blend") -> [w144]
    shift-right: [w106] -> _
    shift-left: 0 -> [w107]
    stop <- _ stop-if-true
    n50 = node-c288() -> ()  [unwired: 1 in, 1 out]
    n51 = Array Size(array=w302) -> (size(s)=w167:i32)
    "sizeArray" <- w167
    n52 = Tick Count (ms)() -> (millisecond timer value=w314:u32)
    "currentTime" <- w314
    n53 = local read "Rva [cmH2O/l/s]"() -> (w253:u8)
    n54 = local read "Cst [ml/cmH2O]"() -> (w252:u8)
    n55 = local read "startSimu"() -> (w102:bool)
    n56 = local read "graphPressure"() -> (w320:dbl)
    n57 = local read "currentTime"() -> (w313:u32)
    n58 = local read "scaleTrigger"() -> (w306:bool)
    n59 = local read "trigger"() -> (w103:bool)
    n60 = local read "scaleTrigger"() -> (w305:bool)
    n61 = local read "scenTrigger"() -> (w134:bool)
    n62 = local read "scenTrigger"() -> (w130:bool)
    n63 = local read "countCycle"() -> (w303:dbl)
    n64 = local read "simuTime"() -> (w344:u8)
    n65 = local read "runBtn"() -> (w143:bool)
    n66 = local read "ventMode"() -> (w174:enum32{"VCV", "PCV"})
    n67 = local read "rstModel"() -> (w250:bool)
    n68 = local read "timeRef1"() -> (w260:dbl)
    n69 = local read "timeRef2"() -> (w259:dbl)
    n70 = local read "timeRef3"() -> (w300:dbl)
    n71 = local read "Cenários"() -> (w132:u16)
    n72 = local read "rstModel"() -> (w251:bool)
    n73 = local read "Cenários"() -> (w135:u16)
    n74 = local read "Cenários"() -> (w131:u16)
    n75 = local read "rstModel"() -> (w249:bool)
    n76 = local read "runBtn"() -> (w349:bool)
    n77 = local read "runBtn"() -> (w341:bool)
    n78 = local read "trigger"() -> (w105:bool)
    n79 = local read "flag1"() -> (w261:bool)
    n80 = local read "flag2"() -> (w262:bool)
    n81 = local read "flag3"() -> (w301:bool)
    n82 = Or(x=w103, y=w102) -> (x .or. y?=w101:bool)
    n83 = Not(x=w143) -> (.not. x?=w142:bool)
    n84 = mathscript code="%flow\nC = C * 0.001;\nx = (C/((R*C)+Ts));\ny = ((R*C)/((R*C)+Ts));\nfK = (x * pK) - (x * pK_1) + (y * fK_1);\n\n%integrator - volume\nvK = vK_1 + ((fK * 60) / 6.0);\n\nif ((runSimu == false) || (rstModel == true))\n  fK = 0; pK = 0; vK = 0;\n  fK_1 = 0; pK_1 = 0; vK_1 = 0;\nend" "lung_model"("pK"=w320, "Ts"=0.01, "R"="Rva [cmH2O/l/s]", "C"="Cst [ml/cmH2O]", "fK_1"=w362, "pK_1"=w316, "vK_1"=w361, "runSimu"=w341, "rstModel"=w251) -> ("fK"=w248:dbl, "pK"=w317:dbl, "vK"=w353:dbl)  [unwired: 1 in, 1 out]
    n85 = case shown="\"PCV\"" w174 {
      tunnel: w314 -> [w6367 w8696]
      tunnel: w368 -> [w6366 w8702]
      tunnel: w367 -> [w6365 w8701]
      tunnel: w366 -> [w6364 w8700]
      tunnel: [w6277 w8687] -> w315
      tunnel: [w6363 w8704] -> w345
      tunnel: w263 -> [w6362 w8705]
      tunnel: [w6361 w8699] -> w365
      tunnel: [w6360 w8698] -> w364
      tunnel: [w6359 w8697] -> w363
      tunnel: [w6274 w8686] -> w326
      tunnel: [w6358 w8685] -> w327
      tunnel: w253 -> [w6357 w8695]
      tunnel: w252 -> [w6356 w8694]
      tunnel: w360 -> [w6355 w8690]
      tunnel: [w6354 w8684] -> w153
      tunnel: w359 -> [w6353 w8689]
      tunnel: [w6352 w8683] -> w152
      tunnel: w358 -> [w6351 w8688]
      tunnel: [w6350 w8682] -> w151
      tunnel: [w6349 w8681] -> w150
      tunnel: [w6348 w8680] -> w332
      tunnel: [w6347 w8679] -> w149
      tunnel: [w6346 w8678] -> w330
      tunnel: [w6345 w8649] -> w148
      tunnel: [w6344 w8658] -> w147
      tunnel: [w6343 w8655] -> w146
      tunnel: [w6342 w8653] -> w145
      tunnel: [w6341 w8677] -> w246
      tunnel: w353 -> [w6340 w8693]
      tunnel: w354 -> [w6322 w8676]
      tunnel: [w6339 w8640] -> w325
      tunnel: "runBtn" -> [w6321 w8647]
      tunnel: [w6338 w8675] -> w347
      tunnel: w346 -> [w6337 w8674]
      tunnel: w248 -> [w6336 w8673]
      tunnel: "enbPalv" -> [w6335 w8645]
      tunnel: [w6334 w8639] -> w324
      tunnel: "enbPmus" -> [w6333 w8646]
      tunnel: "stimBtn" -> [w6332 w8632]
      tunnel: [w6331 w8638] -> w338
      tunnel: w337 -> [w6330 w8641]
      tunnel: w336 -> [w6329 w8643]
      tunnel: [w6328 w8637] -> w335
      tunnel: w334 -> [w6327 w8628]
      tunnel: w333 -> [w6326 w8627]
      tunnel: w331 -> [w6325 w8631]
      tunnel: w329 -> [w6324 w8625]
      tunnel: w305 -> [w6320 w8633]
      tunnel: w281 -> [w6319 _]
      tunnel: [w6318 w8672] -> w280
      tunnel: [w6317 w8672] -> w279
      tunnel: [w6316 w8672] -> w278
      tunnel: [w6315 w8672] -> w277
      tunnel: [w6314 w8672] -> w276
      tunnel: [w6313 w8672] -> w275
      tunnel: [w6312 w8672] -> w274
      tunnel: [w6311 w8672] -> w273
      tunnel: [w6310 w8636] -> w272
      tunnel: w271 -> [w6309 _]
      tunnel: w270 -> [w6308 _]
      tunnel: w269 -> [w6307 _]
      tunnel: w268 -> [w6306 _]
      tunnel: w267 -> [w6305 _]
      tunnel: w266 -> [w6304 _]
      tunnel: w265 -> [w6303 _]
      tunnel: w264 -> [w6302 w8642]
      tunnel: w258 -> [w6301 w8630]
      tunnel: [w6300 w8629] -> w126
      tunnel: [w6299 w8672] -> w257
      tunnel: [w6298 w8672] -> w256
      tunnel: w255 -> [w6297 _]
      tunnel: w254 -> [w6296 _]
      tunnel: w249 -> [w6295 w8634]
      tunnel: "Pausa Inspiratória [s]" -> [w6293 w8670]
      tunnel: "Pmus [cmH2O]" -> [w6292 w8635]
      tunnel: [w6284 w8662] -> w96
      tunnel: w144 -> [w6285 _]
      frame "VCV", Default {
        n86 = local read "flagTime1"() -> (w6281:bool)
        n87 = local read "vcv_volume"() -> (w6291:i16)
        n88 = local read "trigger"() -> (w6282:bool)
        n89 = local read "vcv_peep"() -> (w6288:i16)
        n90 = local read "vcv_flow"() -> (w6290:i16)
        n91 = local read "vcv_sens"() -> (w6287:dbl)
        n92 = local read "vcv_freq"() -> (w6289:i16)
        n93 = local read "vcv_fio2"() -> (w6286:i16)
        n94 = local read "highPeak"() -> (w6265:i16)
        n95 = Or(x=w6282, y=w6281) -> (x .or. y?=w6283:bool)
        n96 = case shown="True" w6283 {
          tunnel: w6285 -> [_ w6378]
          tunnel: [w6368 w6378] -> w6284
          frame True {
            n97 = local read "Cenários"() -> (w6371:u16)
            n98 = Equal?(x=w6371, y=u64 1 ("lower bound (0)")) -> (x = y?=w6369:bool)
            n99 = case shown="True" w6369 {
              tunnel: [w6372 w6377] -> w6368
              frame False {
                n100 = local read "vcv_fio2"() -> (w6372:i16)
              }
              frame True {
                w6373 = u64 15 ("upper bound (100)")
                n101 = local read "vcv_fio2"() -> (w6375:i16)
                n102 = Add(x=w6373, y=w6375) -> (x+y=w6376:u64)
                n103 = Subtract(x=w6375, y=w6373) -> (x-y=w6374:u64)
                n104 = call-poly <vilib>:"Random Number (Range).vi"("lower bound (0)"=w6374, "upper bound (100)"=w6376) -> ("number"=w6377:u64)  [unwired: 9 in]
              }
            }
          }
          frame False {
          }
        }
        n105 = local read "flagTime2"() -> (w6272:bool)
        n106 = local read "flagTime3"() -> (w6271:bool)
        n107 = local read "Cenários"() -> (w6264:u16)
        n108 = mathscript code="Tinsp = (VT / flow) * 60; %inspiration time\nTexp = (60000 / freq) - Tinsp - (inspHold * 1000) + (expHold * 1000); %expiration time\n\nPr = (flow * R) / 60; %resistance pressure\nPe = (VT / C); %elastic pressure \nPIP = Pr + Pe + peep; %peak inspiratory pressure\n\nif (gt(inspHold, 0)) %plateau and driving pressure\n  drivingPressure = (VTI / C);\n  Pplateau = drivingPressure + peep;\nelse\n  Pplateau = 0; drivingPressure = 0;\nend\n\nPEEP = peep; %peep\nFLOW = flow; %flow\n\nrawVolume = rawVolume - (C * peep); %subtract the dead zone volume\nrawFlow = rawFlow * 60; %L/s to L/min\n\nswitch statusVCV\ncase 0 %VCV_INIT\n%parameters\nR = screenR;\nC = screenC;\nVT= screenVT;\nflow = screenFlow;\nfreq = screenFreq;\npeep = screenPeep;\ninspHold = screenInspHold;\nexpHold = screenExpHold;\nsensValue = screenSensValue;\npmusValue = screenPmusValue;\n\ngraphPressure = 0;\n\nstartExpirationTime = time;\nstatusVCV = 1;\n\ncase 1 %VCV_EXPIRATION\nif (gt(inspHold, 0))\n  if (le(time - startExpirationTime, 150))\n      graphPressure = (Pe + peep) - ((Pe * (time - startExpirationTime)) / 150);\n  else\n    graphPressure = peep;\n  end\nelse\n  if (le(time - startExpirationTime, 150))\n    if (scen == 4)\n      graphPressure = peep;\n    else\n      graphPressure = PIP - ((PIP - peep) * ((time - startExpirationTime) / 150));\n    end\n  else \n    graphPressure = peep;\n  end\nend\n\n%sensibility activated\nif ((sensibility == true) && (gt(time - startExpirationTime, 200)))\n  startSensibilityTime = time;\n  flagSens = true;\nend\n\n%fall of pressure\nif ((flagSens == true) && (le(time - startSensibilityTime, sensDuration))) \n  graphPressure = peep + ((sensValue * (time - startSensibilityTime)) / sensDuration);\nend\n\n%end of expiration time (neg)\nif ((flagSens == true) && (gt(time - startSensibilityTime, sensDuration)) && (gt(pmusValue, sensValue*(-1))))\n  expirationTime = (time - startExpirationTime) * 0.001;\n  %frequency = 60 / (inspirationTime + expirationTime);\n  ieRelation = (expirationTime / inspirationTime);\n  VTE = VTI - rawVolume;\n\n  %frequecy filter\n  freqFiltered(rem(countCycle, 5)+1) = (60 / (inspirationTime + expirationTime));\n  frequency = 0;\n  for k = 1:5\n    frequency = frequency + freqFiltered(k);\n  end\n  frequency = frequency * 0.2;\n\n  countCycle = countCycle + 1;\n  startInspirationTime = time;\n  statusVCV = 2;\nend\n\n%end of expiration time\nif (gt(time - startExpirationTime, Texp))\n  expirationTime = (Texp * 0.001);\n  frequency = 60000 / (Tinsp + Texp);\n  ieRelation = (Texp / Tinsp);\n  VTE = VTI - rawVolume;\n  PEEP = graphPressure;\n\n  %frequecy filter\n  freqFiltered(rem(countCycle, 5)+1) = (60000 / (Tinsp + Texp));\n  frequency = 0;\n  for k = 1:5\n    frequency = frequency + freqFiltered(k);\n  end\n  frequency = frequency * 0.2;\n\n  countCycle = countCycle + 1;\n\n  %new parameters\n  R = screenR;\n  C = screenC;\n  VT= screenVT;\n  flow = screenFlow;\n  freq = screenFreq;\n  peep = screenPeep;\n  inspHold = screenInspHold;\n  expHold = screenExpHold;\n  sensValue = screenSensValue;\n  pmusValue = screenPmusValue;\n\n  if (gt(expHold, 0))\n    startHoldTime = time;\n    statusVCV = 4;\n  else\n    startInspirationTime = time;\n    statusVCV = 2;\n  end\nend\n\ncase 2 %VCV_INSPIRATION\nif (le(time - startInspirationTime, Tinsp))\n  graphPressure = (Pr + peep) + ((Pe * (time - startInspirationTime)) / Tinsp);\nelse\n  graphPressure = PIP;\nend\n\nrawFlow = flow;\n\n%end inspiration time\nif (gt(time - startInspirationTime, Tinsp) || ge(graphPressure, highPeak))\n  inspirationTime = Tinsp * 0.001;\n  VTI = rawVolume;  \n  VE = (VTI * 0.001) * frequency;\n  \n  flagSens = false;\n\n  if (gt(inspHold, 0))\n    startHoldTime = time;\n    statusVCV = 3;\n  else\n    startExpirationTime = time;\n    statusVCV = 1;\n  end\nend\n\ncase 3 %INSP_HOLD\ngraphPressure = Pe + peep;\nrawFlow = 0;\n\n%end inspiration hold\nif (gt(time - startHoldTime, inspHold * 1000))\n  startExpirationTime = time;\n  statusVCV = 1;\nend\n\ncase 4 %EXP_HOLD\ngraphPressure = peep;\nrawFlow = 0;\n\n%end expiration hold\nif (gt(time - startHoldTime, expHold * 1000))\n  startInspirationTime = time;\n  statusVCV = 2;\nend\n\nend\n\n%monitoring data default in the first cycle\nif (le(countCycle, 1))\n  VTI = 0; VTE = 0; VE = 0;\n  inspirationTime = 0; expirationTime = 0;\n  frequency  = 0; PEEP = 0; PIP = 0;\n  Pplateau = 0; drivingPressure = 0;\n  FLOW = 0; irRelation = 0; \nend\n\n%plot graphs\nif (runSimu == true)\ngraphVolume = rawVolume; %[mL]\ngraphFlow = rawFlow; %[L/min]\n\nif (statusPmus == true)\n  if ((le(time - startSensibilityTime, sensDuration * 2)) && (flagSens == true))\n    graphPmus = (-1) * pmusValue * sin(((time - startSensibilityTime) / (sensDuration * 2)) * pi);\n  else\n    graphPmus = 0;\n  end\nelse \n  graphPmus = NaN;\nend\n\nif (statusPalv == true)\n  graphAlveolar = ((rawVolume + (20 * peep)) / C);\nelse\n  graphAlveolar = NaN;\nend\n\nend\n\n%re-initialize mode when time scale change\nif ((scaleTrigger == true) || (rstModel == true))\n  statusVCV = 0;\nend\n\n%simulation off\nif (runSimu == false)\n  statusVCV = 0;\n  countCycle = 0;\n\n  VTI = 0; VTE = 0; VE = 0;\n  inspirationTime = 0; expirationTime = 0;\n  frequency = 0; PEEP = 0; PIP = 0;\n  Pplateau = 0; drinvingPressure = 0; \n  FLOW = 0; ieRelation = 0;\n\n  graphVolume = 0; graphFlow = 0; graphPressure = 0;\n  graphAlveolar = 0; graphPmus = 0;\nend" "VCV_mode"("screenVT"=w6291, "screenFlow"=w6290, "screenFreq"=w6289, "screenPeep"=w6288, "time"=w6367, "statusVCV"=w6362, "startExpirationTime"=w6365, "startInspirationTime"=w6366, "screenInspHold"=w6293, "startHoldTime"=w6364, "screenSensValue"=w6287, "screenExpHold"=0.0, "screenFio2"=w6286, "rawVolume"=w6340, "rawFlow"=w6336, "screenR"=w6357, "screenC"=w6356, "VTI"=w6355, "VTE"=w6353, "VE"=w6351, "runSimu"=w6321, "countCycle"=w6337, "statusPalv"=w6335, "statusPmus"=w6333, "sensibility"=w6332, "startSensibilityTime"=w6330, "flagSens"=w6329, "inspirationTime"=w6327, "expirationTime"=w6326, "frequency"=w6325, "ieRelation"=w6324, "sensDuration"=150.0, "screenPmusValue"=w6292, "FLOW"=w6322, "scaleTrigger"=w6320, "VT"=w6319, "flow"=w6309, "freq"=w6308, "peep"=w6307, "inspHold"=w6306, "expHold"=w6305, "sensValue"=w6304, "fio2"=w6303, "pmusValue"=w6302, "freqFiltered"=w6301, "R"=w6297, "C"=w6296, "rstModel"=w6295, "highPeak"=w6265, "scen"=w6264) -> ("statusVCV"=w6363:i32, "startExpirationTime"=w6360:dbl, "startInspirationTime"=w6359:dbl, "graphPressure"=w6275:dbl, "startHoldTime"=w6361:dbl, "graphVolume"=w6358:dbl, "graphFlow"=w6273:dbl, "VTI"=w6354:dbl, "VTE"=w6352:dbl, "VE"=w6350:dbl, "inspirationTime"=w6349:dbl, "expirationTime"=w6348:dbl, "frequency"=w6347:dbl, "ieRelation"=w6346:dbl, "PEEP"=w6345:dbl, "PIP"=w6344:dbl, "Pplateau"=w6343:dbl, "drivingPressure"=w6342:dbl, "FLOW"=w6341:dbl, "graphAlveolar"=w6339:dbl, "countCycle"=w6338:dbl, "graphPmus"=w6334:dbl, "startSensibilityTime"=w6331:dbl, "flagSens"=w6328:bool, "VT"=w6318:dbl, "flow"=w6317:dbl, "freq"=w6316:dbl, "peep"=w6315:dbl, "inspHold"=w6314:dbl, "expHold"=w6313:dbl, "sensValue"=w6312:dbl, "fio2"=w6311:dbl, "pmusValue"=w6310:dbl, "freqFiltered"=w6300:dbl[], "R"=w6299:dbl, "C"=w6298:dbl)  [unwired: 1 in, 1 out]
        n109 = local read "Bat. %"() -> (w6280:u8)
        n110 = Or(x=w6272, y=w6271) -> (x .or. y?=w6270:bool)
        n111 = Less Or Equal?(x=w6280, y=u8 5) -> (x <= y?=w6269:bool)
        n112 = Equal?(x=w6264, y=u8 2) -> (x = y?=w6267:bool)
        n113 = Compound Arithmetic op=AND(w6270, w6269, w6267) -> (w6268:bool)
        n114 = Select(t=0.0, s=w6268, f=w6275) -> (s? t:f=w6277:dbl)
        n115 = Select(t=2.0, s=w6268, f=w6273) -> (s? t:f=w6274:dbl)
      }
      frame "PCV" {
        w8672 = 0.0 ("VT")
        n116 = local read "pcv_blend"() -> (w8663:i8)
        n117 = local read "pcv_tinsp"() -> (w8668:dbl)
        n118 = local read "pcv_peep"() -> (w8665:i16)
        n119 = local read "pcv_sens"() -> (w8664:dbl)
        n120 = local read "pcv_freq"() -> (w8667:i16)
        n121 = local read "pcv_rise"() -> (w8666:dbl)
        n122 = local read "pcv_pc"() -> (w8669:i16)
        n123 = local read "flagTime1"() -> (→"flagTime1 2":bool)
        n124 = local read "flagTime2"() -> (w8623:bool)
        n125 = local read "Cenários"() -> (w8624:u16)
        n126 = mathscript code="Tinsp = (Tinsp * 1000); %inspiration time\nTexp = (60000 / freq) - Tinsp - (inspHold * 1000) + (expHold * 1000); %expiration time\n\ninspirationTime = (Tinsp * 0.001); %inspiration time in seconds\nexpirationTime = (Texp * 0.001); %expiration time in seconds\nfrequency = 60 / (inspirationTime + expirationTime); %frequency\nieRelation = Texp / Tinsp; %i.e relation\npeakPressure = PC + peep;\n\nif (gt(inspHold, 0)) %plateau and driving pressure\n  drivingPressure = (VTI / C);\n  Pplateau = drivingPressure + peep;\nelse\n  Pplateau = 0; drivingPressure = 0;\nend\n\nrawVolume = rawVolume - (20 * peep); %subtract the dead zone volume\nrawFlow = rawFlow * 60; %L/s to L/min\n\nswitch statusPCV\ncase 0 %PCV_INIT\nstartExpirationTime = time;\nstatusPCV = 1;\n\npmusValue = screenPmusValue;\n\ncase 1 %PCV_EXPIRATION\nif (gt(inspHold, 0))\n  if (le(time - startExpirationTime, 0.1 * 1000)) %rise time = 100\n    graphPressure = Pplateau - ((drivingPressure * (time - startExpirationTime)) / (0.1 * 1000));\n  else\n    graphPressure = peep;\n  end\nelse\n  if (le(time - startExpirationTime, 0.1 * 1000))\n    graphPressure = PC - ((PC * (time - startExpirationTime)) / (0.1 * 1000)) + peep;\n  else\n    graphPressure = peep;\n  end\nend\n\n%sensibility activated\nif ((sensibility == true) && (gt(time - startExpirationTime, 200)))\n  startSensibilityTime = time;\n  flagSens = true;\nend\n\n%sensibility activated (scen 5(\nif (gt(time - startExpirationTime, 200) && scen ==5 && flagTime1 == true)\n  startSensibilityTime = time;\n  flagSens = true;\nend\n\n%fall of pressure\nif ((flagSens == true) && (le(time - startSensibilityTime, sensDuration))) \n  if (scen == 5)\n  graphPressure = peep;\n  else\n  graphPressure = peep + ((sens * (time - startSensibilityTime)) / sensDuration);\n  end\nend\n\n%end of expiration time (neg)\nif ((flagSens == true) && (gt(time - startSensibilityTime, sensDuration)) && (gt(pmusValue, sens*(-1))))\n  expirationTime = (time - startExpirationTime) * 0.001;\n  %frequency = 60 / (inspirationTime + expirationTime);\n  ieRelation = (expirationTime / inspirationTime);\n  VTE = VTI - rawVolume;\n\n  %frequecy filter\n  freqFiltered(rem(countCycle, 5)+1) = (60 / (inspirationTime + expirationTime));\n  frequency = 0;\n  for k = 1:5\n    frequency = frequency + freqFiltered(k);\n  end\n  frequency = frequency * 0.2;\n\n  countCycle = countCycle + 1;\n  startInspirationTime = time;\n  statusPCV = 2;\nend\n\n%end of expiration time\nif (gt(time - startExpirationTime, Texp))\n  VTE = VTI - rawVolume;\n  countCycle = countCycle + 1;\n\n  %frequecy filter\n  freqFiltered(rem(countCycle, 5)+1) = (60 / (inspirationTime + expirationTime));\n  frequency = 0;\n  for k = 1:5\n    frequency = frequency + freqFiltered(k);\n  end\n  frequency = frequency * 0.2;\n\n  %new params\n  sensValue = sens;\n  pmusValue = screenPmusValue;\n\n  if (gt(expHold, 0))\n    startHoldTime = time;\n    statusPCV = 4;  \n  else\n    startInspirationTime = time;\n    statusPCV = 2;\n  end\nend\n\ncase 2 %PCV_INSPIRATION\nif (le(time - startInspirationTime, riseTime * 1000))\n  graphPressure = peep + ((PC * (time - startInspirationTime)) / (riseTime * 1000));\nelse\n  if (le(time - startInspirationTime, (riseTime + 0.05) * 1000))\n  graphPressure = PC + peep + 2; \n  else\n  graphPressure = PC + peep;\n  end\nend\n\n%peak flow\nif (gt(rawFlow, peakFlow))\n  peakFlow = rawFlow;\nend\n\n%end inspiration time\nif (gt(time - startInspirationTime, Tinsp))\n  VTI = rawVolume;  \n  VE = (VTI * 0.001) * freq;\n\n  flagSens = false;\n\n  if (gt(inspHold, 0))\n    startHoldTime = time;\n    statusPCV = 3;\n  else\n    startExpirationTime = time;\n    statusPCV = 1;\n  end\nend\n\ncase 3 %INSP_HOLD\ngraphPressure = Pplateau;\nrawFlow = 0;\n\n%end inspiration hold\nif (gt(time - startHoldTime, inspHold * 1000))\n  startExpirationTime = time;\n  statusPCV = 1;\nend\n\ncase 4 %EXP_HOLD\ngraphPressure = peep;\nrawFlow = 0;\n\n%end expiration hold\nif (gt(time - startHoldTime, expHold * 1000))\n  startInspirationTime = time;\n  statusPCV = 2;\nend\n\nend\n\n%graphs\ngraphVolume = rawVolume; %[mL]\ngraphFlow = rawFlow; %[L/min]\n\nif (statusPmus == true)\n  if ((le(time - startSensibilityTime, sensDuration * 2)) && (flagSens == true))\n    graphPmus = (-1) * pmusValue * sin(((time - startSensibilityTime) / (sensDuration * 2)) * pi);\n  else\n    graphPmus = 0;\n  end\nelse \n  graphPmus = NaN;\nend\n\nif (statusPalv == true)\n  graphAlveolar = ((rawVolume + (20 * peep)) / C);\nelse\n  graphAlveolar = NaN;\nend\n\n%re-initialize mode when time scale change\nif ((scaleTrigger == true) || (rstModel == true))\n  statusVCV = 0;\nend\n\n%simulation off\nif (runSimu == false)\n  statusVCV = 0;\n  countCycle = 0;\n\n  VTI = 0; VTE = 0; VE = 0;\n  inspirationTime = 0; expirationTime = 0;\n  frequency = 0; peep = 0; peakPressure = 0;\n  Pplateau = 0; drinvingPressure = 0; \n  peakFlow = 0; ieRelation = 0; Fio2 = 0;\n\n  graphVolume = 0; graphFlow = 0; graphPressure = 0;\n  graphAlveolar = 0; graphPmus = 0;\nend" "PCV_mode"("statusPCV"=w8705, "PC"=w8669, "peep"=w8665, "Tinsp"=w8668, "freq"=w8667, "inspHold"=w8670, "expHold"=0.0, "sens"=w8664, "Fio2"=w8663, "riseTime"=w8666, "graphVolume"=0.0 ("rawPressure"), "startInspirationTime"=w8702, "startExpirationTime"=w8701, "startHoldTime"=w8700, "time"=w8696, "R"=w8695, "C"=w8694, "rawVolume"=w8693, "rawFlow"=w8673, "graphFlow"=0.0, "graphPressure"=0.0, "VTI"=w8690, "VTE"=w8689, "VE"=w8688, "peakFlow"=w8676, "countCycle"=w8674, "runSimu"=w8647, "statusPmus"=w8646, "statusPalv"=w8645, "sensDuration"=150.0 ("sensDurantion"), "pmusValue"=w8642, "flagSens"=w8643, "startSensibilityTime"=w8641, "screenPmusValue"=w8635, "rstModel"=w8634, "scaleTrigger"=w8633, "sensibility"=w8632, "frequency"=w8631, "freqFiltered"=w8630, "inspirationTime"=w8628, "expirationTime"=w8627, "ieRelation"=w8625, "scen"=w8624, "flagTime1"=w8623) -> ("statusPCV"=w8704:i32, "startInspirationTime"=w8697:dbl, "startExpirationTime"=w8698:dbl, "startHoldTime"=w8699:dbl, "graphPressure"=w8687:dbl, "graphFlow"=w8686:dbl, "graphVolume"=w8685:dbl, "VTI"=w8684:dbl, "VTE"=w8683:dbl, "VE"=w8682:dbl, "inspirationTime"=w8681:dbl, "expirationTime"=w8680:dbl, "frequency"=w8679:dbl, "peep"=w8648:i32, "peakPressure"=w8659:i32, "ieRelation"=w8678:dbl, "peakFlow"=w8677:dbl, "Pplateau"=w8656:dbl, "drivingPressure"=w8652:dbl, "countCycle"=w8675:dbl, "Fio2"=w8662:i32, "graphAlveolar"=w8640:dbl, "graphPmus"=w8639:dbl, "pmusValue"=w8636:dbl, "flagSens"=w8637:bool, "startSensibilityTime"=w8638:dbl, "freqFiltered"=w8629:dbl[])  [unwired: 1 in, 1 out]
        n127 = local read "Cenários"() -> (w8626:u16)
        n128 = Equal?(x=w8626, y=u16 3) -> (x = y?=w8650:bool)
        n129 = Select(t=0.0, s=w8650, f=w8659) -> (s? t:f=w8658:dbl)
        n130 = Select(t=0.0, s=w8650, f=w8656) -> (s? t:f=w8655:dbl)
        n131 = Select(t=0.0, s=w8650, f=w8652) -> (s? t:f=w8653:dbl)
        n132 = Select(t=0.0, s=w8650, f=w8648) -> (s? t:f=w8649:dbl)
      }
    }
    "graphPressure" <- w315
    "countCycle" <- w347
    "vti" <- w153
    "ve" <- w151
    "pPeak" <- w147
    "PEEP" <- w148
    "vte" <- w152
    "tInsp" <- w150
    "fTotal" <- w149
    "pPlateau" <- w146
    "drivingP" <- w145
    "pFlow" <- w246
    "Fio2" <- w96
    n133 = mathscript code="if (runSimu == true)\ngraphTime = (currentTime - (initTime + ((scale * 1000) * count))) * 0.001;\n\nindex = index + 1;\nvec_1(index) = graphTime;\nvec_2(index) = volume;\nvec_3(index) = flow;\n\nif (scen == 3)\nvec_4(index) = 0;\nelse\nvec_4(index) = Paw;\nend\n\nvec_5(index) = Palv;\nvec_6(index) = Pmus;\nvec_10(index) = 0;\n\nfor k = (index+1):(index+25)\nvec_2(k) = NaN; vec_3(k) = NaN;\nvec_4(k) = NaN; vec_5(k) = NaN;\nvec_6(k) = NaN;\nend\n\nif (gt(graphTime, scale))\n  count = count + 1;\n  index = 0;\n  trigger = true;\nend\n\n%during the first second, clean graph\nif (eq(count, 0))\n  if (le(graphTime, 1))\n    vec_2(index) = NaN; vec_3(index) = NaN;\n    vec_4(index) = NaN; vec_5(index) = NaN;\n    vec_6(index) = NaN;\n  end\nend\n\nend\n\nif (runSimu == false)\n\nif (flag1 == true)\n  for k = 1:arraySize\n    if (vec_1(k) == timeRef1)\n      indexRef = k;\n    end\n  end\nend\n\nif (flag2 == true)\n  for k = 1:arraySize\n    if (vec_1(k) == timeRef2)\n      indexRef = k;\n    end\n  end\nend\n\nif (flag3 == true)\n  for k = 1:arraySize\n    if (vec_1(k) == timeRef3)\n      indexRef = k;\n    end\n  end\nend\n\nif (gt((currentTime - initClock) - cleanCursor, 10))\n  cleanCursor = (currentTime - initClock);\n  for k = 0:arraySize\n    vec_7(k+1) = -2000; \n    vec_8(k+1) = -2000; \n    vec_9(k+1) = -2000;\n  end\nend\n\nif ((flag1 == true) || (flag2 == true) || (flag3 == true))\n  vec_7(indexRef) = 2000; \n  vec_8(indexRef) = 2000; \n  vec_9(indexRef) = 2000;\nend\n\nif ((flag1 == false) && (flag2 == false) && (flag3 == false))\n  indexRef = 1;\nend\n\nend\n\n%clean graphs when time scale change\nif (scaleTrigger == true)\n  initTime = currentTime;\n  graphTime = 0;\n  count = 0;\n  index = 0;\n\n  for k = 1:arraySize\n    vec_1(k) = NaN; vec_2(k) = NaN; vec_3(k) = NaN;\n    vec_4(k) = NaN; vec_5(k) = NaN; vec_6(k) = NaN;\n    vec_7(k) = NaN; vec_8(k) = NaN; vec_9(k) = NaN;\n  end\nend\n\nif ((runSimu == false) || (rstModel == true))\n  initTime = currentTime;\n  graphTime = 0;\n  count = 0;\n  index = 0;\nend" "base_time"("initTime"=w348, "count"=w352, "currentTime"=w313, "scale"=w344, "runSimu"=w349, "volume"=w327, "flow"=w326, "Palv"=w325, "Paw"=w315, "Pmus"=w324, "vec_1"=w302, "vec_2"=w175, "vec_3"=w179, "vec_4"=w178, "vec_5"=w176, "vec_6"=w177, "index"=w323, "arraySize"=w167, "trigger"=FALSE, "scaleTrigger"=w306, "flag1"=w261, "flag2"=w262, "flag3"=w301, "timeRef1"=w260, "timeRef2"=w259, "timeRef3"=w300, "indexRef"=w299, "vec_7"=w298, "vec_8"=w297, "vec_9"=w296, "cleanCursor"=w291, "initClock"=w290, "rstModel"=w250, "scen"=w132) -> ("count"=w351:dbl, "initTime"=w350:u32, "vec_1"=w173:dbl[], "vec_2"=w168:dbl[], "vec_3"=w170:dbl[], "vec_4"=w169:dbl[], "vec_5"=w322:dbl[], "vec_6"=w236:dbl[], "index"=w120:dbl, "trigger"=w119:bool, "indexRef"=w288:dbl, "vec_7"=w289:dbl[], "vec_8"=w284:dbl[], "vec_9"=w282:dbl[], "cleanCursor"=w292:dbl)  [unwired: 1 in, 1 out]
    "trigger" <- w119
    "indexRef" <- w288
    n134 = case shown="True" w101 {
      tunnel: [w4033 "Tempo de Simulação [s]"] -> w208
      tunnel: w311 -> [w4033 _]
      tunnel: w303 -> [_ w4034]
      frame False {
      }
      frame True {
        n135 = local read "pPeak"() -> (w4043:i16)
        n136 = local read "minFlow"() -> (w4061:dbl)
        n137 = local read "pFlow"() -> (w4042:i16)
        n138 = local read "Pmus [cmH2O]"() -> (w4063:dbl)
        n139 = local read "vti"() -> (w4044:i16)
        n140 = Absolute Value(x=w4043) -> (abs(x)=w4056:i16)
        n141 = local read "enbPmus"() -> (w4064:bool)
        n142 = Absolute Value(x=w4061) -> (abs(x)=w4062:dbl)
        n143 = Divide(x=w4044, y=50.0) -> (x/y=w4059:dbl)
        n144 = Round To Nearest(number=w4056) -> (nearest integer value=w4055:i16)
        n145 = Round To Nearest(number=w4042) -> (nearest integer value=w4050:i16)
        n146 = Quotient & Remainder(x=w4055, y=10.0) -> (x-y*floor(x/y)=w4054:dbl, floor(x/y)=w4053:dbl)
        n147 = Quotient & Remainder(x=w4050, y=10.0) -> (x-y*floor(x/y)=w4049:dbl, floor(x/y)=w4048:dbl)
        n148 = Round To Nearest(number=w4062) -> (nearest integer value=w4057:dbl)
        n149 = Round To Nearest(number=w4059) -> (nearest integer value=w4058:dbl)
        n150 = mathscript code="if (gt(countCycle, 1))\n%pressure\nif (gt(restP, 5))\n  upperLimitP = (numP * 10) + 10;\nelse\n  upperLimitP = (numP * 10) + 5;\nend\n\nif (statusPmus == true)\n  lowerLimitP = (-1) * (pmusValue + 2);\nelse\n  lowerLimitP = 0;\nend\n\n%flow\nif (gt(restF, 5)) \n  upperLimitF = (numF * 10) + 15;\nelse\n  upperLimitF = (numF * 10) + 10;\nend\n\nif (gt(negF, 0))\n  lowerLimitF = (-1) * (negF + 5);\nelse\n  lowerLimitF = -90;\nend\n\n%volume\nif (gt(numV, 0))\n  upperLimitV = (numV + 1) * 50;\nelse\n  upperLimitV = 500;\nend\nlowerLimitV = 0;\n\nelse\n  upperLimitV = 500; lowerLimitV = 0;\n  upperLimitF = 40; lowerLimitF = -90;\n  upperLimitP = 40; lowerLimitP = 0;\nend"("restP"=w4054, "countCycle"=w4034, "statusPmus"=w4064, "pmusValue"=w4063, "numV"=w4058, "restF"=w4049, "negF"=w4057, "numP"=w4053, "numF"=w4048) -> ("upperLimitP"=w4039:dbl, "lowerLimitP"=w4040:dbl, "upperLimitF"=w4038:dbl, "lowerLimitF"=w4037:dbl, "upperLimitV"=w4036:dbl, "lowerLimitV"=w4035:i32)  [unwired: 1 in, 1 out]
        n151 = property on="graph4" class="XYGraph (strict)"("YScale.Maximum"=w4036, "YScale.Minimum"=w4035) -> ()  [unwired: 2 in, 2 out]
        n152 = property on="graph4" class="XYGraph (strict)"("XScale.Maximum"=w4039) -> ()  [unwired: 2 in, 2 out]
        n153 = property on="graph5" class="XYGraph (strict)"("YScale.Maximum"=w4038, "YScale.Minimum"=w4037) -> ()  [unwired: 2 in, 2 out]
        n154 = property on="graph5" class="XYGraph (strict)"("XScale.Maximum"=w4036, "XScale.Minimum"=w4035) -> ()  [unwired: 2 in, 2 out]
        n155 = property on="graph3" class="XYGraph (strict)"("YScale.Maximum"=w4039, "YScale.Minimum"=w4040) -> ()  [unwired: 2 in, 2 out]
        n156 = property on="graph2" class="XYGraph (strict)"("YScale.Maximum"=w4038, "YScale.Minimum"=w4037) -> ()  [unwired: 2 in, 2 out]
        n157 = property on="graph1" class="XYGraph (strict)"("YScale.Maximum"=w4036, "YScale.Minimum"=w4035) -> ()  [unwired: 2 in, 2 out]
        n158 = property on="graph1" class="XYGraph (strict)"("XScale.Maximum"="Tempo de Simulação [s]") -> ()  [unwired: 2 in, 2 out]
        n159 = property on="graph2" class="XYGraph (strict)"("XScale.Maximum"="Tempo de Simulação [s]") -> ()  [unwired: 2 in, 2 out]
        n160 = property on="graph3" class="XYGraph (strict)"("XScale.Maximum"="Tempo de Simulação [s]") -> ()  [unwired: 2 in, 2 out]
        n161 = property on="StringVolume" class="Str"("Visible"=FALSE) -> ()  [unwired: 2 in, 2 out]
        n162 = property on="StringFlow" class="Str"("Visible"=FALSE) -> ()  [unwired: 2 in, 2 out]
        n163 = property on="StringPressure" class="Str"("Visible"=FALSE) -> ()  [unwired: 2 in, 2 out]
      }
    }
    "simuTime" <- w208
    n164 = event shown="[1] \"graph1\": Mouse Move" {
      selector: _ -> [_ _ _ _]
      dyn-events: _ -> [_ _ _ _]
      timeout: 1 -> [_ _ _ _]
      tunnel: w175 -> [_ w3702 w3815 w3926]
      tunnel: w179 -> [_ w3704 w3813 w3925]
      tunnel: w178 -> [_ w3703 w3814 w3924]
      tunnel: w177 -> [_ w3700 w3811 w3922]
      tunnel: w176 -> [_ w3701 w3812 w3923]
      event Timeout {
        n165 = event-data() -> ()  [unwired: 1 in, 3 out]
      }
      event "graph1": Mouse Move {
        n166 = event-data() -> ("Coords"=w3706:T9)  [unwired: 1 in, 4 out]
        n167 = local read "runBtn"() -> (w3707:bool)
        n168 = Not(x=w3707) -> (.not. x?=w3705:bool)
        n169 = case shown="True" w3705 {
          tunnel: w3706 -> [_ w3796]
          tunnel: w3704 -> [_ w3743]
          tunnel: w3703 -> [_ w3740]
          tunnel: w3702 -> [_ w3747]
          tunnel: w3701 -> [_ w3728]
          tunnel: w3700 -> [_ w3727]
          frame False {
          }
          frame True {
            n170 = local read "indexRef"() -> (w3726:dbl)
            n171 = invoke on="graph1" class="XYGraph (strict)" method="GetPlotAtPos"("InputPt"=w3796) -> ("PlotNum"=w3797:i32)  [unwired: 4 in, 4 out]
            n172 = invoke on="graph1" class="XYGraph (strict)" method="Map Coords To XY"("Coords"=w3796) -> ("XY"=w3802:cluster{"X":dbl, "Y":dbl})  [unwired: 6 in, 6 out]
            n173 = Index Array(array=w3728, index=w3726) -> (element=w3751:dbl)
            n174 = Index Array(array=w3727, index=w3726) -> (element=w3750:dbl)
            n175 = Not Equal?(x=-1, y=w3797) -> (x != y?=w3710:bool)
            "flag1" <- w3710
            n176 = Unbundle(w3802) -> ("X"=w3735:dbl)  [unwired: 1 out]
            n177 = Number To Fractional String(number=w3751, precision (6)=i16 2) -> (F-format string=w3760:string)  [unwired: 2 in]
            n178 = Number To Fractional String(number=w3750, precision (6)=i16 2) -> (F-format string=w3752:string)  [unwired: 2 in]
            n179 = Equal?(x=w3760, y="NaN") -> (x = y?=w3758:bool)
            n180 = Equal?(x=w3752, y="NaN") -> (x = y?=w3754:bool)
            n181 = Multiply(x=w3735, y=100.0) -> (x*y=w3792:dbl)
            n182 = Select(t="-", s=w3754, f=w3752) -> (s? t:f=w3755:string)
            n183 = Select(t="-" ("string"), s=w3758, f=w3760) -> (s? t:f=w3761:string)
            n184 = Unbundle(w3796) -> ("Horizontal"=w3800:i32, "Vertical"=w3801:i32)
            n185 = Round To Nearest(number=w3792) -> (nearest integer value=w3791:dbl)
            n186 = Index Array(array=w3747, index=w3726) -> (element=w3746:dbl)
            n187 = Index Array(array=w3743, index=w3726) -> (element=w3744:dbl)
            n188 = Index Array(array=w3740, index=w3726) -> (element=w3741:dbl)
            n189 = Add(x=10, y=w3800) -> (x+y=w3736:i32)
            n190 = Multiply(x=w3791, y=0.01) -> (x*y=→"timeRef1":dbl)
            n191 = Bundle(w3736, "Vertical"=w3801) -> (w3737:cluster{i32, "Vertical":i32})  [unwired: 1 in]
            n192 = Concatenate Strings("Pmus: " ("string"), w3755, " [cmH2O]" ("string"), "\r\n") -> (w3764:string)
            n193 = Concatenate Strings("Palv: " ("string"), w3761, " [cmH2O]" ("string"), "\r\n") -> (w3769:string)
            n194 = Number To Fractional String(number=w3746, precision (6)=i16 2) -> (F-format string=w3807:string)  [unwired: 2 in]
            n195 = Number To Fractional String(number=w3735, precision (6)=i16 2) -> (F-format string=w3803:string)  [unwired: 2 in]
            n196 = Number To Fractional String(number=w3744, precision (6)=i16 2) -> (F-format string=w3787:string)  [unwired: 2 in]
            n197 = Number To Fractional String(number=w3735, precision (6)=i16 2) -> (F-format string=w3783:string)  [unwired: 2 in]
            n198 = Number To Fractional String(number=w3741, precision (6)=i16 2) -> (F-format string=w3780:string)  [unwired: 2 in]
            n199 = Number To Fractional String(number=w3735, precision (6)=i16 2) -> (F-format string=w3732:string)  [unwired: 2 in]
            n200 = local read "enbPmus"() -> (w3714:bool)
            n201 = local read "enbPalv"() -> (w3715:bool)
            n202 = Select(t=w3769, s=w3715, f="") -> (s? t:f=w3731:string)
            n203 = Select(t=w3764, s=w3714, f="") -> (s? t:f=w3730:string)
            n204 = Concatenate Strings("Tempo: " ("string"), w3732, " [s]" ("string")) -> (w3729:string)
            n205 = Boolean To (0,1)(Boolean=w3715) -> (0, 1=w3717:i16)
            n206 = Boolean To (0,1)(Boolean=w3714) -> (0, 1=w3716:i16)
            n207 = Concatenate Strings("Volume: " ("string"), w3807, " [ml]" ("string"), "\r\n", "Tempo: " ("string"), w3803, " [s]" ("string")) -> (w3795:string)
            n208 = Concatenate Strings("Fluxo: " ("string"), w3787, " [l/min]" ("string"), "\r\n", "Tempo: " ("string"), w3783, " [s]" ("string")) -> (w3776:string)
            n209 = Concatenate Strings("Paw: " ("string"), w3780, " [cmH2O]" ("string"), "\r\n", w3731, w3730, w3729) -> (w3775:string)
            n210 = Not Equal To 0?(x=w3717) -> (x != 0?=w3725:bool)
            n211 = Not Equal To 0?(x=w3716) -> (x != 0?=w3722:bool)
            n212 = Select(t=15.0, s=w3725, f=0.0) -> (s? t:f=w3719:dbl)
            n213 = Select(t=15.0, s=w3722, f=0.0) -> (s? t:f=w3718:dbl)
            n214 = Add(x=w3719, y=w3718) -> (x+y=w3713:dbl)
            n215 = Bundle(w3736, u32 1340) -> (w3739:cluster{i32, u32})  [unwired: 1 in]
            n216 = Bundle(w3736, u32 1536) -> (w3738:cluster{i32, u32})  [unwired: 1 in]
            n217 = Add(x=35.0, y=w3713) -> (x+y=w3712:dbl)
            n218 = property on="StringPressure" class="Str"("Height"=w3712) -> ()  [unwired: 2 in, 2 out]
            n219 = property on="StringVolume" class="Str"("Visible"=w3710, "Position"=w3737, "Value"=w3795) -> ()  [unwired: 2 in, 2 out]
            n220 = property on="StringFlow" class="Str"("Visible"=w3710, "Position"=w3739, "Value"=w3776) -> ()  [unwired: 2 in, 2 out]
            n221 = property on="StringPressure" class="Str"("Visible"=w3710, "Position"=w3738, "Value"=w3775) -> ()  [unwired: 2 in, 2 out]
            n222 = property on="flag2" class="Bool (strict)"("Value"=FALSE) -> ()  [unwired: 2 in, 2 out]
            n223 = property on="flag3" class="Bool (strict)"("Value"=FALSE) -> ()  [unwired: 2 in, 2 out]
          }
        }
      }
      event "graph2": Mouse Move {
        n224 = event-data() -> ("Coords"=w3817:T9)  [unwired: 1 in, 4 out]
        n225 = local read "runBtn"() -> (w3818:bool)
        n226 = Not(x=w3818) -> (.not. x?=w3816:bool)
        n227 = case shown="True" w3816 {
          tunnel: w3817 -> [_ w3907]
          tunnel: w3815 -> [_ w3879]
          tunnel: w3814 -> [_ w3877]
          tunnel: w3813 -> [_ w3878]
          tunnel: w3812 -> [_ w3842]
          tunnel: w3811 -> [_ w3841]
          frame False {
          }
          frame True {
            n228 = local read "indexRef"() -> (w3837:dbl)
            n229 = invoke on="graph2" class="XYGraph (strict)" method="GetPlotAtPos"("InputPt"=w3907) -> ("PlotNum"=w3909:i32)  [unwired: 4 in, 4 out]
            n230 = invoke on="graph2" class="XYGraph (strict)" method="Map Coords To XY"("Coords"=w3907) -> ("XY"=w3913:cluster{"X":dbl, "Y":dbl})  [unwired: 6 in, 6 out]
            n231 = Index Array(array=w3842, index=w3837) -> (element=w3848:dbl)
            n232 = Index Array(array=w3841, index=w3837) -> (element=w3847:dbl)
            n233 = Not Equal?(x=-1, y=w3909) -> (x != y?=w3821:bool)
            "flag2" <- w3821
            n234 = Unbundle(w3913) -> ("X"=w3873:dbl)  [unwired: 1 out]
            n235 = Number To Fractional String(number=w3848, precision (6)=i16 2) -> (F-format string=w3858:string)  [unwired: 2 in]
            n236 = Number To Fractional String(number=w3847, precision (6)=i16 2) -> (F-format string=w3850:string)  [unwired: 2 in]
            n237 = Equal?(x=w3858, y="NaN") -> (x = y?=w3856:bool)
            n238 = Equal?(x=w3850, y="NaN") -> (x = y?=w3852:bool)
            n239 = Unbundle(w3907) -> ("Horizontal"=w3912:i32, "Vertical"=w3886:i32)
            n240 = Multiply(x=w3873, y=100.0) -> (x*y=w3897:dbl)
            n241 = Select(t="-", s=w3852, f=w3850) -> (s? t:f=w3853:string)
            n242 = Select(t="-" ("string"), s=w3856, f=w3858) -> (s? t:f=w3859:string)
            n243 = Add(x=10, y=w3912) -> (x+y=w3838:i32)
            n244 = Round To Nearest(number=w3897) -> (nearest integer value=w3896:dbl)
            n245 = Index Array(array=w3879, index=w3837) -> (element=w3876:dbl)
            n246 = Index Array(array=w3878, index=w3837) -> (element=w3875:dbl)
            n247 = Index Array(array=w3877, index=w3837) -> (element=w3874:dbl)
            n248 = Multiply(x=w3896, y=0.01) -> (x*y=→"timeRef2":dbl)
            n249 = Bundle(w3838, "Vertical"=w3886) -> (w3839:cluster{i32, "Vertical":i32})  [unwired: 1 in]
            n250 = Concatenate Strings("Pmus: " ("string"), w3853, " [cmH2O]" ("string"), "\r\n") -> (w3862:string)
            n251 = Number To Fractional String(number=w3876, precision (6)=i16 2) -> (F-format string=w3904:string)  [unwired: 2 in]
            n252 = Number To Fractional String(number=w3873, precision (6)=i16 2) -> (F-format string=w3900:string)  [unwired: 2 in]
            n253 = Number To Fractional String(number=w3875, precision (6)=i16 2) -> (F-format string=w3918:string)  [unwired: 2 in]
            n254 = Number To Fractional String(number=w3873, precision (6)=i16 2) -> (F-format string=w3914:string)  [unwired: 2 in]
            n255 = Number To Fractional String(number=w3874, precision (6)=i16 2) -> (F-format string=w3890:string)  [unwired: 2 in]
            n256 = Number To Fractional String(number=w3873, precision (6)=i16 2) -> (F-format string=w3870:string)  [unwired: 2 in]
            n257 = Concatenate Strings("Palv: " ("string"), w3859, " [cmH2O]" ("string"), "\r\n") -> (w3867:string)
            n258 = local read "enbPmus"() -> (w3823:bool)
            n259 = local read "enbPalv"() -> (w3824:bool)
            n260 = Select(t=w3867, s=w3824, f="") -> (s? t:f=w3845:string)
            n261 = Select(t=w3862, s=w3823, f="") -> (s? t:f=w3844:string)
            n262 = Concatenate Strings("Tempo: " ("string"), w3870, " [s]" ("string")) -> (w3843:string)
            n263 = Boolean To (0,1)(Boolean=w3824) -> (0, 1=w3828:i16)
            n264 = Boolean To (0,1)(Boolean=w3823) -> (0, 1=w3827:i16)
            n265 = Concatenate Strings("Volume: " ("string"), w3904, " [ml]" ("string"), "\r\n", "Tempo: " ("string"), w3900, " [s]" ("string")) -> (w3899:string)
            n266 = Concatenate Strings("Fluxo: " ("string"), w3918, " [l/min]" ("string"), "\r\n", "Tempo: " ("string"), w3914, " [s]" ("string")) -> (w3908:string)
            n267 = Concatenate Strings("Paw: " ("string"), w3890, " [cmH2O]" ("string"), "\r\n", w3845, w3844, w3843) -> (w3887:string)
            n268 = Not Equal To 0?(x=w3828) -> (x != 0?=w3836:bool)
            n269 = Not Equal To 0?(x=w3827) -> (x != 0?=w3833:bool)
            n270 = Select(t=15.0, s=w3836, f=0.0) -> (s? t:f=w3830:dbl)
            n271 = Select(t=15.0, s=w3833, f=0.0) -> (s? t:f=w3829:dbl)
            n272 = Add(x=w3830, y=w3829) -> (x+y=w3826:dbl)
            n273 = Bundle(w3838, u32 1142) -> (w3880:cluster{i32, u32})  [unwired: 1 in]
            n274 = Bundle(w3838, u32 1536) -> (w3840:cluster{i32, u32})  [unwired: 1 in]
            n275 = Add(x=35.0, y=w3826) -> (x+y=w3822:dbl)
            n276 = property on="StringVolume" class="Str"("Visible"=w3821, "Position"=w3880, "Value"=w3899) -> ()  [unwired: 2 in, 2 out]
            n277 = property on="StringFlow" class="Str"("Visible"=w3821, "Position"=w3839, "Value"=w3908) -> ()  [unwired: 2 in, 2 out]
            n278 = property on="StringPressure" class="Str"("Visible"=w3821, "Position"=w3840, "Value"=w3887) -> ()  [unwired: 2 in, 2 out]
            n279 = property on="StringPressure" class="Str"("Height"=w3822) -> ()  [unwired: 2 in, 2 out]
            n280 = property on="flag3" class="Bool (strict)"("Value"=FALSE) -> ()  [unwired: 2 in, 2 out]
            n281 = property on="flag1" class="Bool (strict)"("Value"=FALSE) -> ()  [unwired: 2 in, 2 out]
          }
        }
      }
      event "graph3": Mouse Move {
        n282 = event-data() -> ("Coords"=w3927:T9)  [unwired: 1 in, 4 out]
        n283 = local read "runBtn"() -> (w3929:bool)
        n284 = Not(x=w3929) -> (.not. x?=w3928:bool)
        n285 = case shown="True" w3928 {
          tunnel: w3927 -> [_ w4021]
          tunnel: w3926 -> [_ w3966]
          tunnel: w3925 -> [_ w3965]
          tunnel: w3924 -> [_ w3964]
          tunnel: w3923 -> [_ w3950]
          tunnel: w3922 -> [_ w3949]
          frame False {
          }
          frame True {
            n286 = local read "indexRef"() -> (w3948:dbl)
            n287 = invoke on="graph3" class="XYGraph (strict)" method="GetPlotAtPos"("InputPt"=w4021) -> ("PlotNum"=w4022:i32)  [unwired: 4 in, 4 out]
            n288 = invoke on="graph3" class="XYGraph (strict)" method="Map Coords To XY"("Coords"=w4021) -> ("XY"=w4027:cluster{"X":dbl, "Y":dbl})  [unwired: 6 in, 6 out]
            n289 = Index Array(array=w3950, index=w3948) -> (element=w3952:dbl)
            n290 = Index Array(array=w3949, index=w3948) -> (element=w3951:dbl)
            n291 = Not Equal?(x=-1, y=w4022) -> (x != y?=w3932:bool)
            "flag3" <- w3932
            n292 = Unbundle(w4027) -> ("X"=w3960:dbl)  [unwired: 1 out]
            n293 = Number To Fractional String(number=w3952, precision (6)=i16 2) -> (F-format string=w3983:string)  [unwired: 2 in]
            n294 = Number To Fractional String(number=w3951, precision (6)=i16 2) -> (F-format string=w3975:string)  [unwired: 2 in]
            n295 = Equal?(x=w3983, y="NaN") -> (x = y?=w3981:bool)
            n296 = Equal?(x=w3975, y="NaN") -> (x = y?=w3977:bool)
            n297 = Unbundle(w4021) -> ("Horizontal"=w4025:i32, "Vertical"=w4026:i32)
            n298 = Multiply(x=w3960, y=100.0) -> (x*y=w4018:dbl)
            n299 = Select(t="-", s=w3977, f=w3975) -> (s? t:f=w3978:string)
            n300 = Select(t="-" ("string"), s=w3981, f=w3983) -> (s? t:f=w3984:string)
            n301 = Add(x=10, y=w4025) -> (x+y=w3961:i32)
            n302 = Round To Nearest(number=w4018) -> (nearest integer value=w4017:dbl)
            n303 = Index Array(array=w3966, index=w3948) -> (element=w3969:dbl)
            n304 = Index Array(array=w3965, index=w3948) -> (element=w3970:dbl)
            n305 = Index Array(array=w3964, index=w3948) -> (element=w3968:dbl)
            n306 = Multiply(x=w4017, y=0.01) -> (x*y=→"timeRef3":dbl)
            n307 = Bundle(w3961, "Vertical"=w4026) -> (w3962:cluster{i32, "Vertical":i32})  [unwired: 1 in]
            n308 = Number To Fractional String(number=w3969, precision (6)=i16 2) -> (F-format string=w4015:string)  [unwired: 2 in]
            n309 = Number To Fractional String(number=w3960, precision (6)=i16 2) -> (F-format string=w4011:string)  [unwired: 2 in]
            n310 = Number To Fractional String(number=w3970, precision (6)=i16 2) -> (F-format string=w4004:string)  [unwired: 2 in]
            n311 = Number To Fractional String(number=w3960, precision (6)=i16 2) -> (F-format string=w4000:string)  [unwired: 2 in]
            n312 = Concatenate Strings("Pmus: " ("string"), w3978, " [cmH2O]" ("string"), "\r\n") -> (w3987:string)
            n313 = Number To Fractional String(number=w3968, precision (6)=i16 2) -> (F-format string=w4030:string)  [unwired: 2 in]
            n314 = Number To Fractional String(number=w3960, precision (6)=i16 2) -> (F-format string=w3953:string)  [unwired: 2 in]
            n315 = Concatenate Strings("Palv: " ("string"), w3984, " [cmH2O]" ("string"), "\r\n") -> (w3992:string)
            n316 = local read "enbPmus"() -> (w3933:bool)
            n317 = local read "enbPalv"() -> (w3934:bool)
            n318 = Select(t=w3992, s=w3934, f="") -> (s? t:f=w3956:string)
            n319 = Select(t=w3987, s=w3933, f="") -> (s? t:f=w3955:string)
            n320 = Concatenate Strings("Tempo: " ("string"), w3953, " [s]" ("string")) -> (w3954:string)
            n321 = Boolean To (0,1)(Boolean=w3934) -> (0, 1=w3939:i16)
            n322 = Boolean To (0,1)(Boolean=w3933) -> (0, 1=w3938:i16)
            n323 = Concatenate Strings("Volume: " ("string"), w4015, " [ml]" ("string"), "\r\n", "Tempo: " ("string"), w4011, " [s]" ("string")) -> (w3999:string)
            n324 = Concatenate Strings("Fluxo: " ("string"), w4004, " [l/min]" ("string"), "\r\n", "Tempo: " ("string"), w4000, " [s]" ("string")) -> (w3997:string)
            n325 = Concatenate Strings("Paw: " ("string"), w4030, " [cmH2O]" ("string"), "\r\n", w3956, w3955, w3954) -> (w3963:string)
            n326 = Not Equal To 0?(x=w3939) -> (x != 0?=w3947:bool)
            n327 = Not Equal To 0?(x=w3938) -> (x != 0?=w3944:bool)
            n328 = Select(t=15.0, s=w3947, f=0.0) -> (s? t:f=w3941:dbl)
            n329 = Select(t=15.0, s=w3944, f=0.0) -> (s? t:f=w3940:dbl)
            n330 = Add(x=w3941, y=w3940) -> (x+y=w3937:dbl)
            n331 = Bundle(w3961, u32 1142) -> (w3973:cluster{i32, u32})  [unwired: 1 in]
            n332 = Bundle(w3961, u32 1340) -> (w3974:cluster{i32, u32})  [unwired: 1 in]
            n333 = Add(x=35.0, y=w3937) -> (x+y=w3935:dbl)
            n334 = property on="flag1" class="Bool (strict)"("Value"=FALSE) -> ()  [unwired: 2 in, 2 out]
            n335 = property on="flag2" class="Bool (strict)"("Value"=FALSE) -> ()  [unwired: 2 in, 2 out]
            n336 = property on="StringVolume" class="Str"("Visible"=w3932, "Position"=w3973, "Value"=w3999) -> ()  [unwired: 2 in, 2 out]
            n337 = property on="StringFlow" class="Str"("Visible"=w3932, "Position"=w3974, "Value"=w3997) -> ()  [unwired: 2 in, 2 out]
            n338 = property on="StringPressure" class="Str"("Visible"=w3932, "Position"=w3962, "Value"=w3963) -> ()  [unwired: 2 in, 2 out]
            n339 = property on="StringPressure" class="Str"("Height"=w3935) -> ()  [unwired: 2 in, 2 out]
          }
        }
      }
    }
    n340 = mathscript code="vcv_volume = volume;\nvcv_flow = flow;\nvcv_freq = freq;\nvcv_peep = peep;\nvcv_sens = sens;\nvcv_blend = blend;\n\n%volume\nif (ge(vcv_volume, 1000))\nif (vol_up == true)\nvcv_volume = volume + 100;\nend\nif (vol_down == true)\nvcv_volume = volume - 100;\nend\nelse \nif (vol_up == true)\nvcv_volume = volume + 10;\nend\nif (vol_down == true)\nvcv_volume = volume - 10;\nend\nend\n\nif (gt(vcv_volume, 2000))\nvcv_volume = 2000;\nend\n\nif (le(vcv_volume, 0))\nvcv_volume = 0;\nend\n\n%flow\nif (flow_up == true)\nvcv_flow = flow + 1;\nend\n\nif (flow_down == true)\nvcv_flow = flow - 1;\nend\n\nif (gt(vcv_flow, 50))\nvcv_flow = 50;\nend\n\nif (le(vcv_flow, 1))\nvcv_flow = 1;\nend\n\n%freq\nif (freq_up == true)\nvcv_freq = freq + 1;\nend\n\nif (freq_down == true)\nvcv_freq = freq - 1;\nend\n\nif (gt(vcv_freq, 50))\nvcv_freq = 50;\nend\n\nif (le(vcv_freq, 1))\nvcv_freq = 1;\nend\n\n%peep\nif (peep_up == true)\nvcv_peep = peep + 1;\nend\n\nif (peep_down == true)\nvcv_peep = peep - 1;\nend\n\nif (gt(vcv_peep, 20))\nvcv_peep = 20;\nend\n\nif (le(vcv_peep, 0))\nvcv_peep = 0;\nend\n\n%sens\nif (sens_up == true)\nvcv_sens = sens + 0.1;\nend\n\nif (sens_down == true)\nvcv_sens = sens - 0.1;\nend\n\nif (gt(vcv_sens, 15))\nvcv_sens = 15;\nend\n\nif (le(vcv_sens, -15))\nvcv_sens = -15;\nend\n\n%blend\nif (blend_up == true)\nvcv_blend = blend + 1;\nend\n\nif (blend_down == true)\nvcv_blend = blend - 1;\nend\n\nif (gt(vcv_blend, 100))\nvcv_blend = 100;\nend\n\nif (le(vcv_blend, 21))\nvcv_blend = 21;\nend\n\n\n%CENÁRIOS\nif (trigger == true && scen == 0)\nvcv_volume = 400;\nvcv_flow = 24;\nvcv_freq = 20;\nvcv_peep = 5;\nvcv_sens = -3.0;\nvcv_blend = 100;\nend\n\n%1\nif (trigger == true && scen == 1)\nvcv_volume = 450;\nvcv_flow = 27;\nvcv_freq = 20;\nvcv_peep = 5;\nvcv_sens = -1.0;\nvcv_blend = 40;\nend\n\n%2\nif (trigger == true && scen == 2)\nvcv_volume = 350;\nvcv_flow = 15;\nvcv_freq = 15;\nvcv_peep = 6;\nvcv_sens = -2.0;\nvcv_blend = 75;\nend\n\n%4\nif (trigger == true && scen == 4)\nvcv_volume = 430;\nvcv_flow = 26;\nvcv_freq = 15;\nvcv_peep = 5;\nvcv_sens = -1.5;\nvcv_blend = 80;\nend"("volume"=w232, "flow"=w231, "freq"=w230, "peep"=w229, "sens"=w228, "blend"=w227, "vol_up"="volume_up", "vol_down"="volume_down", "flow_up"="flow_up", "flow_down"="flow_down", "freq_up"="freq_up", "freq_down"="freq_down", "peep_up"="peep_up", "peep_down"="peep_down", "sens_up"="sens_up", "sens_down"="sens_down", "blend_up"="vcv_blend_up", "blend_down"="vcv_blend_down", "trigger"=w134, "scen"=w135) -> ("vcv_volume"=w214:i32, "vcv_flow"=w213:i32, "vcv_freq"=w210:i32, "vcv_peep"=w211:i32, "vcv_sens"=w212:dbl, "vcv_blend"=w136:i32)  [unwired: 1 in, 1 out]
    "vcv_volume" <- w214
    "vcv_flow" <- w213
    "vcv_freq" <- w210
    "vcv_peep" <- w211
    "vcv_sens" <- w212
    "vcv_fio2" <- w136
    n341 = mathscript code="pcv_pc = pc;\npcv_tinsp = tinsp;\npcv_freq = freq;\npcv_rise = rise;\npcv_peep = peep;\npcv_sens = sens;\npcv_blend = blend;\n\n%pc\nif (pc_up == true)\npcv_pc = pc + 1;\nend\n\nif (pc_down == true)\npcv_pc = pc - 1;\nend\n\nif (gt(pcv_pc, 50))\npcv_pc = 50;\nend\n\nif (le(pcv_pc, 1))\npcv_pc = 1;\nend\n\n%tinsp\nif (tinsp_up == true)\npcv_tinsp = tinsp + 0.1;\nend\n\nif (tinsp_down == true)\npcv_tinsp = tinsp - 0.1;\nend\n\nif (gt(pcv_tinsp, 5))\npcv_tinsp = 5;\nend\n\nif (le(pcv_tinsp, 0.1))\npcv_tinsp = 0.1;\nend\n\n%freq\nif (freq_up == true)\npcv_freq = freq + 1;\nend\n\nif (freq_down == true)\npcv_freq = freq - 1;\nend\n\nif (gt(pcv_freq, 50))\npcv_freq = 50;\nend\n\nif (le(pcv_freq, 1))\npcv_freq = 1;\nend\n\n%rise time\nif (rise_up == true)\npcv_rise = rise + 0.05;\nend\n\nif (rise_down == true)\npcv_rise = rise - 0.05;\nend\n\nif (gt(pcv_rise, 0.5))\npcv_rise = 0.5;\nend\n\nif (le(pcv_rise, 0))\npcv_rise = 0;\nend\n\n%peep\nif (peep_up == true)\npcv_peep = peep + 1;\nend\n\nif (peep_down == true)\npcv_peep = peep - 1;\nend\n\nif (gt(pcv_peep, 20))\npcv_peep = 20;\nend\n\nif (le(pcv_peep, 0))\npcv_peep = 0;\nend\n\n%sens\nif (sens_up == true)\npcv_sens = sens + 0.1;\nend\n\nif (sens_down == true)\npcv_sens = sens - 0.1;\nend\n\nif (gt(pcv_sens, 15))\npcv_sens = 15;\nend\n\nif (le(pcv_sens, -15))\npcv_sens = -15;\nend\n\n%blend\nif (blend_up == true)\npcv_blend = blend + 1;\nend\n\nif (blend_down == true)\npcv_blend = blend - 1;\nend\n\nif (gt(pcv_blend, 100))\npcv_blend = 100;\nend\n\nif (le(pcv_blend, 21))\npcv_blend = 21;\nend\n\n\n\n%CENÁRIOS\nif (trigger == true && scen == 3)\npcv_pc = 12;\npcv_tinsp = 1;\npcv_freq = 17;\npcv_rise = 0.25;\npcv_peep = 3;\npcv_sens = -2.0;\npcv_blend = 85;\nend\n\nif (trigger == true && scen == 5)\npcv_pc = 12;\npcv_tinsp = 1.2;\npcv_freq = 25;\npcv_rise = 0.05;\npcv_peep = 5;\npcv_sens = -5.0;\npcv_blend = 85;\nend"("pc"=w207, "tinsp"=w206, "freq"=w205, "rise"=w204, "peep"=w203, "sens"=w202, "blend"=w201, "pc_up"="pc_up", "pc_down"="pc_down", "tinsp_up"="tinsp_up", "tinsp_down"="tinsp_down", "freq_up"="freq_up", "freq_down"="freq_down", "rise_up"="rise_up", "rise_down"="rise_down", "peep_up"="peep_up", "peep_down"="peep_down", "sens_up"="sens_up", "sens_down"="sens_down", "blend_up"="blend_up", "blend_down"="blend_down", "scen"=w131, "trigger"=w130) -> ("pcv_pc"=w180:dbl, "pcv_tinsp"=w181:dbl, "pcv_freq"=w182:dbl, "pcv_rise"=w183:dbl, "pcv_peep"=w184:dbl, "pcv_sens"=w185:dbl, "pcv_blend"=w186:dbl)  [unwired: 1 in, 1 out]
    "pcv_pc" <- w180
    "pcv_tinsp" <- w181
    "pcv_freq" <- w182
    "pcv_rise" <- w183
    "pcv_peep" <- w184
    "pcv_sens" <- w185
    "pcv_blend" <- w186
    n342 = case shown="True" w105 {
      tunnel: w166 -> [w1167 w1178]
      tunnel: [w1167 w1177] -> w165
      tunnel: w107 -> [w1166 w1172]
      tunnel: [w1166 w1171] -> w106
      frame False {
      }
      frame True {
        n343 = local read "Bat. %"() -> (w1169:u8)
        n344 = local read "pPeak"() -> (w1203:i16)
        n345 = local read "pFlow"() -> (w1204:i16)
        n346 = local read "fTotal"() -> (w1201:i16)
        n347 = local read "PEEP"() -> (w1202:dbl)
        n348 = local read "Fio2"() -> (w1179:i16)
        n349 = local read "vte"() -> (w1199:i16)
        n350 = local read "vti"() -> (w1198:i16)
        n351 = local read "ve"() -> (w1200:dbl)
        n352 = Less Or Equal?(x=w1169, y=20.0) -> (x <= y?=w1168:bool)
        n353 = mathscript code="alarm = '';\npriority = 0;\ncounter = 0;\n\n%ve\nif (gt(ve,highVe))\nalarm = 'VOLUME MINUTO Alto';\npriority = 1;\ncounter = counter + 1;\nelse\nif (lt(ve,lowVe))\nalarm = 'VOLUME MINUTO Baixo';\npriority = 1;\ncounter = counter + 1;\nend\nend\n\n%peep\nif (gt(peep,highPeep))\nalarm = 'PEEP Alta';\npriority = 1;\ncounter = counter + 1;\nelse\nif (lt(peep,lowPeep))\nalarm = 'PEEP Baixa';\npriority = 1;\ncounter = counter + 1;\nend\nend\n\n%freq\nif (gt(freq,highFreq))\nalarm = 'FREQUÊNCIA Alta';\npriority = 1;\ncounter = counter + 1;\nelse\nif (lt(freq,lowFreq))\nalarm = 'FREQUÊNCIA Baixa';\npriority = 1;\ncounter = counter + 1;\nend\nend\n\n%blend\nif (gt(blend,highBlend))\nalarm = 'FiO2 Alto';\npriority = 1;\ncounter = counter + 1;\nelse\nif (lt(blend,lowBlend))\nalarm = 'FiO2 Baixo';\npriority = 1;\ncounter = counter + 1;\nend\nend\n\n%vti\nif (gt(vti,highVti))\nalarm = 'VOLUME CORRENTE Alto';\npriority = 2;\ncounter = counter + 1;\nelse\nif (lt(vti,lowVti))\nalarm = 'VOLUME CORRENTE Baixo';\npriority = 2;\ncounter = counter + 1;\nend\nend\n\n%vte\nif (gt(vte,highVte))\nalarm = 'VOLUME EXPIRATÓRIO Alto';\npriority = 2;\ncounter = counter + 1;\nelse\nif (lt(vte,lowVte))\nalarm = 'VOLUME EXPIRATÓRIO Baixo';\npriority = 2;\ncounter = counter + 1;\nend\nend\n\n%pPeak\nif (gt(pPeak,highPeak))\nalarm = 'PRESSÃO Alta';\npriority = 2;\ncounter = counter + 1;\nelse\nif (lt(pPeak,lowPeak))\nalarm = 'PRESSÃO Baixa';\npriority = 2;\ncounter = counter + 1;\nend\nend\n\n%flow\nif (gt(pFlow,highFlow))\nalarm = 'FLUXO Alto';\npriority = 2;\ncounter = counter + 1;\nelse\nif (lt(pFlow,lowFlow))\nalarm = 'FLUXO Baixo';\npriority = 2;\ncounter = counter + 1;\nend\nend\n\n%battery\nif (bat_val == true)\nalarm = 'BATERIA fraca'; \npriority = 2;\ncounter = counter + 1;\nend"("highVti"="highVti", "lowVti"="lowVti", "highVte"="highVte", "lowVte"="lowVte", "highVe"="highVe", "lowVe"="lowVe", "highPeak"="highPeak", "lowPeak"="lowPeak", "highPeep"="highPeep", "lowPeep"="lowPeep", "highFreq"="highFreq", "lowFreq"="lowFreq", "highFlow"="highFlow", "lowFlow"="lowFlow", "vti"=w1198, "vte"=w1199, "ve"=w1200, "freq"=w1201, "peep"=w1202, "pPeak"=w1203, "pFlow"=w1204, "highBlend"="highFio2", "lowBlend"="lowFio2", "blend"=w1179, "counter"=w1178, "priority"=w1172, "bat_val"=w1168) -> ("alarm"=w1174:string, "priority"=w1171:i32, "counter"=w1177:i32)  [unwired: 1 in, 1 out]
        n354 = Number To Decimal String(number=w1177) -> (decimal integer string=w1176:string)  [unwired: 1 in]
        n355 = case shown="0, Default" w1171 {
          tunnel: [u32 0 ("Colors:BG Color") u32 0 ("Colors:BG Color") u32 16777225 ("Colors:BG Color")] -> w1182
          tunnel: [u32 0 ("Colors:BG Color") u32 16777022 ("Colors:BG Color") u32 16711680 ("Colors:BG Color")] -> w1183
          frame 0, Default {
          }
          frame 1 {
          }
          frame 2 {
          }
        }
        n356 = Concatenate Strings(w1176, "  ", w1174) -> (→"alarm_text":string)
        n357 = property on="alarm_text" class="Str"("Text.FontColor"=w1182) -> ()  [unwired: 2 in, 2 out]
        n358 = property on="alarm_text" class="Str"("Text.BGColor"=w1183) -> ()  [unwired: 2 in, 2 out]
      }
    }
    n359 = case shown="False" w142 {
      frame False {
        n360 = local read "startSimu"() -> (w674:bool)
        n361 = case shown="True" w674 {
          frame False {
          }
          frame True {
            n362 = property on="Cenários" class="Ring (strict)"("DisabledEnum"=T7."Disabled and Grayed Out" ("Disabled")) -> ()  [unwired: 2 in, 2 out]
          }
        }
      }
      frame True {
        n363 = property on="Cenários" class="Ring (strict)"("DisabledEnum"=T7."Enabled" ("Disabled")) -> ()  [unwired: 2 in, 2 out]
      }
    }
    n364 = local read "scenTrigger"() -> (w137:bool)
    n365 = case shown="True" w137 {
      frame False {
      }
      frame True {
        n366 = local read "Cenários"() -> (w389:u16)
        n367 = property on="Cst [ml/cmH2O]" class="Slide (strict)"("Value"=u8 45 ("Cst [ml/cmH2O]")) -> ()  [unwired: 2 in, 2 out]
        n368 = property on="Rva [cmH2O/l/s]" class="Slide (strict)"("Value"=u8 5 ("Rva [cmH2O/l/s]")) -> ()  [unwired: 2 in, 2 out]
        n369 = case shown="5" w389 {
          frame 0, Default {
            n370 = property on="ventMode" class="TabCtl (strict)"("Value"=enum32{"VCV", "PCV"}."VCV" ("ventMode")) -> ()  [unwired: 2 in, 2 out]
            n371 = property on="highVti" class="DigNum (strict)"("Value"=i16 450 ("highVti")) -> ()  [unwired: 2 in, 2 out]
            n372 = property on="highVte" class="DigNum (strict)"("Value"=i16 450 ("highVte")) -> ()  [unwired: 2 in, 2 out]
            n373 = property on="highFio2" class="DigNum (strict)"("Value"=i16 100 ("highFio2")) -> ()  [unwired: 2 in, 2 out]
            n374 = property on="lowFio2" class="DigNum (strict)"("Value"=i16 21 ("lowFio2")) -> ()  [unwired: 2 in, 2 out]
            n375 = property on="Bat. %" class="Slide (strict)"("Value"=u8 100 ("Bat. %")) -> ()  [unwired: 2 in, 2 out]
          }
          frame 1 {
            w402 = u16 0 items=["Masculino", "Feminino"] ("Sexo")
            n376 = property on="Sexo" class="Ring (strict)"("Value"=w402) -> ()  [unwired: 2 in, 2 out]
            n377 = property on="Idade (anos)" class="DigNum (strict)"("Value"=u8 42 ("Idade (anos)")) -> ()  [unwired: 2 in, 2 out]
            n378 = property on="Altura (m)" class="DigNum (strict)"("Value"=1.8 ("Altura (m)")) -> ()  [unwired: 2 in, 2 out]
            n379 = property on="Peso (kg)" class="DigNum (strict)"("Value"=u16 70 ("Peso (kg)")) -> ()  [unwired: 2 in, 2 out]
            n380 = property on="ventMode" class="TabCtl (strict)"("Value"=enum32{"VCV", "PCV"}."VCV" ("ventMode")) -> ()  [unwired: 2 in, 2 out]
            n381 = property on="highFio2" class="DigNum (strict)"("Value"=i16 45 ("highFio2")) -> ()  [unwired: 2 in, 2 out]
            n382 = property on="lowFio2" class="DigNum (strict)"("Value"=i16 35 ("lowFio2")) -> ()  [unwired: 2 in, 2 out]
            n383 = property on="highVti" class="DigNum (strict)"("Value"=i16 500 ("highVti")) -> ()  [unwired: 2 in, 2 out]
            n384 = property on="highVte" class="DigNum (strict)"("Value"=i16 500 ("highVte")) -> ()  [unwired: 2 in, 2 out]
            n385 = property on="Bat. %" class="Slide (strict)"("Value"=u8 100 ("Bat. %")) -> ()  [unwired: 2 in, 2 out]
          }
          frame 2 {
            n386 = property on="ventMode" class="TabCtl (strict)"("Value"=enum32{"VCV", "PCV"}."VCV" ("ventMode")) -> ()  [unwired: 2 in, 2 out]
            n387 = property on="highVti" class="DigNum (strict)"("Value"=i16 400 ("highVti")) -> ()  [unwired: 2 in, 2 out]
            n388 = property on="highVte" class="DigNum (strict)"("Value"=i16 400 ("highVte")) -> ()  [unwired: 2 in, 2 out]
            n389 = property on="highFlow" class="DigNum (strict)"("Value"=i16 30 ("highFlow")) -> ()  [unwired: 2 in, 2 out]
            n390 = property on="highFio2" class="DigNum (strict)"("Value"=i16 80 ("highFio2")) -> ()  [unwired: 2 in, 2 out]
            n391 = property on="lowFio2" class="DigNum (strict)"("Value"=i16 60 ("lowFio2")) -> ()  [unwired: 2 in, 2 out]
            n392 = property on="highPeak" class="DigNum (strict)"("Value"=i16 35 ("highPeak")) -> ()  [unwired: 2 in, 2 out]
            n393 = property on="lowVti" class="DigNum (strict)"("Value"=i16 200 ("lowVti")) -> ()  [unwired: 2 in, 2 out]
            n394 = property on="lowVte" class="DigNum (strict)"("Value"=i16 200 ("lowVte")) -> ()  [unwired: 2 in, 2 out]
            n395 = property on="Bat. %" class="Slide (strict)"("Value"=u8 80 ("Bat. %")) -> ()  [unwired: 2 in, 2 out]
          }
          frame 3 {
            n396 = property on="ventMode" class="TabCtl (strict)"("Value"=enum32{"VCV", "PCV"}."PCV" ("ventMode")) -> ()  [unwired: 2 in, 2 out]
            n397 = property on="highVti" class="DigNum (strict)"("Value"=i16 300 ("highVti")) -> ()  [unwired: 2 in, 2 out]
            n398 = property on="highVte" class="DigNum (strict)"("Value"=i16 300 ("highVte")) -> ()  [unwired: 2 in, 2 out]
            n399 = property on="highPeak" class="DigNum (strict)"("Value"=i16 20 ("highPeak")) -> ()  [unwired: 2 in, 2 out]
            n400 = property on="highFio2" class="DigNum (strict)"("Value"=i16 100 ("highFio2")) -> ()  [unwired: 2 in, 2 out]
            n401 = property on="highFlow" class="DigNum (strict)"("Value"=i16 100 ("highFlow")) -> ()  [unwired: 2 in, 2 out]
            n402 = property on="lowFio2" class="DigNum (strict)"("Value"=i16 21 ("lowFio2")) -> ()  [unwired: 2 in, 2 out]
            n403 = property on="Bat. %" class="Slide (strict)"("Value"=u8 100 ("Bat. %")) -> ()  [unwired: 2 in, 2 out]
          }
          frame 4 {
            (unwired) u8 15 ("lungC")
            (unwired) u8 10 ("lungR")
            n404 = property on="ventMode" class="TabCtl (strict)"("Value"=enum32{"VCV", "PCV"}."VCV" ("ventMode")) -> ()  [unwired: 2 in, 2 out]
            n405 = property on="Idade (anos)" class="DigNum (strict)"("Value"=u8 65 ("Idade (anos)")) -> ()  [unwired: 2 in, 2 out]
            n406 = property on="Altura (m)" class="DigNum (strict)"("Value"=1.73 ("Altura (m)")) -> ()  [unwired: 2 in, 2 out]
            n407 = property on="Peso (kg)" class="DigNum (strict)"("Value"=u16 72 ("Peso (kg)")) -> ()  [unwired: 2 in, 2 out]
            n408 = property on="highVte" class="DigNum (strict)"("Value"=i16 500 ("highVte")) -> ()  [unwired: 2 in, 2 out]
            n409 = property on="highVti" class="DigNum (strict)"("Value"=i16 500 ("highVti")) -> ()  [unwired: 2 in, 2 out]
            n410 = property on="Bat. %" class="Slide (strict)"("Value"=u8 100 ("Bat. %")) -> ()  [unwired: 2 in, 2 out]
            n411 = property on="Cst [ml/cmH2O]" class="Slide (strict)"("Value"=u8 15 ("Cst [ml/cmH2O]")) -> ()  [unwired: 2 in, 2 out]
            n412 = property on="Rva [cmH2O/l/s]" class="Slide (strict)"("Value"=u8 10 ("Rva [cmH2O/l/s]")) -> ()  [unwired: 2 in, 2 out]
            n413 = property on="highPeak" class="DigNum (strict)"("Value"=i16 30 ("highPeak")) -> ()  [unwired: 2 in, 2 out]
            n414 = property on="highFio2" class="DigNum (strict)"("Value"=i16 100 ("highFio2")) -> ()  [unwired: 2 in, 2 out]
          }
          frame 5 {
            w445 = u16 1 items=["Masculino", "Feminino"] ("Sexo")
            n415 = property on="ventMode" class="TabCtl (strict)"("Value"=enum32{"VCV", "PCV"}."PCV" ("ventMode")) -> ()  [unwired: 2 in, 2 out]
            n416 = property on="Sexo" class="Ring (strict)"("Value"=w445) -> ()  [unwired: 2 in, 2 out]
            n417 = property on="Idade (anos)" class="DigNum (strict)"("Value"=u8 45 ("Idade (anos)")) -> ()  [unwired: 2 in, 2 out]
            n418 = property on="Altura (m)" class="DigNum (strict)"("Value"=1.74 ("Altura (m)")) -> ()  [unwired: 2 in, 2 out]
            n419 = property on="Peso (kg)" class="DigNum (strict)"("Value"=u16 150 ("Peso (kg)")) -> ()  [unwired: 2 in, 2 out]
            n420 = property on="Bat. %" class="Slide (strict)"("Value"=u8 100 ("Bat. %")) -> ()  [unwired: 2 in, 2 out]
            n421 = property on="Rva [cmH2O/l/s]" class="Slide (strict)"("Value"=u8 12 ("Rva [cmH2O/l/s]")) -> ()  [unwired: 2 in, 2 out]
            n422 = property on="enbPmus" class="Bool (strict)"("Value"=TRUE ("enbPmus")) -> ()  [unwired: 2 in, 2 out]
            n423 = property on="Pmus [cmH2O]" class="Slide (strict)"("Value"=1.5 ("Pmus [cmH2O]")) -> ()  [unwired: 2 in, 2 out]
            n424 = property on="highVti" class="DigNum (strict)"("Value"=i16 700 ("highVti")) -> ()  [unwired: 2 in, 2 out]
            n425 = property on="highVte" class="DigNum (strict)"("Value"=i16 700 ("highVte")) -> ()  [unwired: 2 in, 2 out]
            n426 = property on="highVe" class="DigNum (strict)"("Value"=18.0 ("highVe")) -> ()  [unwired: 2 in, 2 out]
            n427 = property on="highFlow" class="DigNum (strict)"("Value"=i16 100 ("highFlow")) -> ()  [unwired: 2 in, 2 out]
          }
        }
      }
    }
    n428 = Bundle("vec_1"=w173, "vec_7"=w289) -> (w295:cluster{"vec_1":dbl[], "vec_7":dbl[]})  [unwired: 1 in]
    n429 = Bundle("vec_1"=w173, "vec_2"=w168) -> (w294:cluster{"vec_1":dbl[], "vec_2":dbl[]})  [unwired: 1 in]
    n430 = Build Array(w295, w294) -> (→"graph1":cluster{"vec_1":dbl[], "vec_2":dbl[]}[])
    n431 = call-poly <vilib>:"Random Number (Range).vi"("lower bound (0)"=u64 0, "upper bound (100)"=u64 500) -> ("number"=w118:u64)  [unwired: 9 in]
    n432 = call-poly <vilib>:"Random Number (Range).vi"("lower bound (0)"=u64 500, "upper bound (100)"=u64 1000) -> ("number"=w117:u64)  [unwired: 9 in]
    n433 = Bundle("vec_1"=w173, "vec_8"=w284) -> (w287:cluster{"vec_1":dbl[], "vec_8":dbl[]})  [unwired: 1 in]
    n434 = Bundle("vec_1"=w173, "vec_3"=w170) -> (w286:cluster{"vec_1":dbl[], "vec_3":dbl[]})  [unwired: 1 in]
    n435 = Array Max & Min(array=w170) -> (max value=→"maxFlow":dbl, min value=→"minFlow":dbl)  [unwired: 2 out]
    n436 = local read "Rva [cmH2O/l/s]"() -> (w242:u8)
    n437 = local read "Cst [ml/cmH2O]"() -> (w241:u8)
    n438 = Build Array(w287, w286) -> (→"graph2":cluster{"vec_1":dbl[], "vec_3":dbl[]}[])
    n439 = local read "ventMode"() -> (w129:enum32{"VCV", "PCV"})
    n440 = local read "trigger"() -> (w104:bool)
    n441 = local read "scenTrigger"() -> (w98:bool)
    n442 = case shown="True" "info" {
      frame False {
      }
      frame True {
        n443 = local read "Cenários"() -> (w377:u16)
        n444 = case shown="5" w377 {
          tunnel: ["SIMULAÇÃO LIVRE!" "Um paciente adulto de 70 kg, previamente estável e em ventilação mecânica controlada, está sendo ventilado com uma fração de oxigênio inspirada (FiO2) de 40%, conforme os parâmetros ajustados no ventilador mecânico. No entanto, a equipe clínica começa a notar discrepâncias nas leituras da FiO2 fornecidas pelo monitor do ventilador. Em alguns momentos, o valor registrado é de 25%, enquanto, em outros, atinge 80%, sem que houvesse ajustes manuais no aparelho.\n\nO paciente não apresenta sinais imediatos de deterioração clínica, mas as leituras permanecem inconsistentes." "Um paciente adulto está recebendo ventilação mecânica no modo VCV através do ventilador. Durante o suporte ventilatório, a equipe clínica observa que o ventilador começa a emitir alertas intermitentes relacionados à energia, sem sinais claros de falha nos parâmetros ventilatórios. Após alguns minutos, a ventilação se torna irregular, com períodos de interrupção no fornecimento do volume respiratório programado.\n\nOs parâmetros configurados, como volume corrente e frequência respiratória, permanecem visíveis e corretos, e o monitor continua registrando outros dados vitais normalmente. No entanto, a ventilação parece estar progressivamente falhando, e a equipe não identifica imediatamente a causa do problema." "Um paciente adulto em ventilação mecânica invasiva está sendo monitorado em um ventilador. Durante a verificação de rotina dos parâmetros do ventilador, a equipe clínica percebe que os valores de pressão das vias aéreas estão ausentes ou não condizem com os padrões esperados. Entretanto, todos os demais parâmetros, como volume corrente, frequência respiratória e saturação de oxigênio, continuam sendo monitorados corretamente e não indicam nenhuma irregularidade aparente.\n\nApesar da ausência de leitura adequada de pressão, o paciente parece clinicamente estável, sem sinais de desconforto respiratório imediato." "Paciente idoso, com histórico de Silicose, foi admitido na Unidade de Terapia Intensiva devido a um quadro de Insuficiência Respiratória Aguda (IrpA). A Silicose, por causar fibrose pulmonar, resultou em um distúrbio ventilatório restritivo, caracterizado por dificuldades respiratórias progressivas. O paciente também evoluiu com falência renal e, nas últimas 24 horas, apresentou um balanço hídrico positivo de +4000 ml, não sendo capaz de tolerar Terapia de Substituição Renal (TSR).\n\nOs exames gasométricos mostram:\n- pH: 7,48\n- HCO3: 34 mEq/L\n- PaO2: 61 mmHg\n- SaO2: 89%\n\nNa monitorização ventilatória, os parâmetros são:\n- Cst: 15 ml/cmH2O\n- Elastância: 61 cmH2O/L\n- Pplat: 45 cmH2O" "Paciente obesa, tabagista e asmática, em desmame de drogas sedativas e bloqueador neuromuscular devido ventilação difícil, evoluindo com má adaptação na VM (assincronia paciente-ventilador).\n\n"] -> w378
          frame 0, Default {
          }
          frame 1 {
          }
          frame 2 {
          }
          frame 3 {
          }
          frame 4 {
          }
          frame 5 {
          }
        }
        n445 = call "Display Message to User"("Message"=w378) -> ()  [unwired: 9 in, 2 out]
      }
    }
    n446 = mathscript code="pred = 0;\n\nif (sexo == 0)\npred = 50 + (0.91 * ((altura * 100) - 152.4));\nelse\npred = 45.5 + (0.91 * ((altura * 100) - 152.4));\nend\n\n\ncoef = 1;\nsat = 0;\nX = 0;\nY = 0;\n\nif (sexo == 0)\nif (le(idade, 30))\ncoef = 1.3;\nX = 1;\nend\n\nif (gt(idade, 30) && le(idade, 40) && X == 0)\ncoef = 1.2;\nX = 1;\nend\n\nif (gt(idade, 40) && le(idade, 50) && X == 0)\ncoef = 1.1;\nX = 1;\nend\n\nif (gt(idade, 50) && le(idade, 60) && X == 0)\ncoef = 1.07;\nX = 1;\nend\n\nif (X == 0)\ncoef = 1;\nend\n\nelse \nif (le(idade, 30))\ncoef = 1.4;\nY = 1;\nend\n\nif (gt(idade, 30) && le(idade, 40) && Y == 0)\ncoef = 1.3;\nY = 1;\nend\n\nif (gt(idade, 40) && le(idade, 50) && Y == 0)\ncoef = 1.1;\nY = 1;\nend\n\nif (gt(idade, 50) && le(idade, 60) && Y == 0)\ncoef = 1.05;\nY = 1;\nend\n\nif (Y == 0)\ncoef = 0.95;\nend\nend\n\nsat = 97 - ((freqC - 80) / coef)"("sexo"="Sexo", "idade"="Idade (anos)", "altura"="Altura (m)", "peso"="Peso (kg)", "freqC"=90.0) -> ("pred"=→"Peso Ideal (kg)":dbl, "sat"=w158:dbl)  [unwired: 1 in, 1 out]
    n447 = case shown="True" w104 {
      frame False {
      }
      frame True {
        n448 = local read "Cenários"() -> (w376:u16)
        n449 = local read "Bat. %"() -> (w371:u8)
        n450 = Subtract(x=w371, y=30.0) -> (x-y=w372:dbl)
        n451 = Equal?(x=w376, y=u16 2) -> (x = y?=w373:bool)
        n452 = Select(t=w372, s=w373, f=w371) -> (s? t:f=→"Bat. %":dbl)
      }
    }
    n453 = feedback-in #1(w242) -> ()
    n454 = feedback #1() -> (w244:u8)  [unwired: 1 in]
    n455 = feedback #2() -> (w243:u8)  [unwired: 1 in]
    n456 = feedback-in #2(w241) -> ()
    n457 = feedback-in #3(w129) -> ()
    n458 = feedback #3() -> (w128:enum32{"VCV", "PCV"})  [unwired: 1 in]
    n459 = local read "Tempo de Simulação [s]"() -> (w209:u8)
    n460 = Not Equal?(x=w242, y=w244) -> (x != y?=w240:bool)
    n461 = Not Equal?(x=w241, y=w243) -> (x != y?=w239:bool)
    n462 = Not Equal?(x=w129, y=w128) -> (x != y?=w99:bool)
    n463 = Or(x=w240, y=w239) -> (x .or. y?=w238:bool)
    n464 = Bundle("vec_1"=w173, "vec_9"=w282) -> (w283:cluster{"vec_1":dbl[], "vec_9":dbl[]})  [unwired: 1 in]
    n465 = Bundle("vec_1"=w173, "vec_4"=w169) -> (w328:cluster{"vec_1":dbl[], "vec_4":dbl[]})  [unwired: 1 in]
    n466 = Bundle("vec_1"=w173, "vec_5"=w322) -> (w343:cluster{"vec_1":dbl[], "vec_5":dbl[]})  [unwired: 1 in]
    n467 = Bundle("vec_1"=w173, "vec_6"=w236) -> (w340:cluster{"vec_1":dbl[], "vec_6":dbl[]})  [unwired: 1 in]
    n468 = local read "trigger"() -> (w237:bool)
    n469 = local read "simuTime"() -> (w310:u8)
    n470 = local read "trigger"() -> (w308:bool)
    n471 = Build Array(w283, w328, w343, w340) -> (→"graph3":cluster{"vec_1":dbl[], "vec_6":dbl[]}[])
    n472 = And(x=w238, y=w237) -> (x .and. y?=w100:bool)
    n473 = Not Equal?(x=w209, y=w310) -> (x != y?=w309:bool)
    n474 = Compound Arithmetic op=OR(w100, w99, w98) -> (→"rstModel":bool)
    n475 = And(x=w309, y=w308) -> (x .and. y?=→"scaleTrigger":bool)
    n476 = feedback #4() -> (w138:u16)  [unwired: 1 in]
    n477 = feedback-in #4("Cenários") -> ()
    n478 = Bundle("vec_4"=w169, "vec_2"=w168) -> (→"graph4":cluster{"vec_4":dbl[], "vec_2":dbl[]})  [unwired: 1 in]
    n479 = Not Equal?(x="Cenários", y=w138) -> (x != y?=→"scenTrigger":bool)
    n480 = Number To Fractional String(number=w330, precision (6)=i16 1) -> (F-format string=w356:string)  [unwired: 2 in]
    n481 = local read "rstModel"() -> (w127:bool)
    n482 = Concatenate Strings("1:", w356) -> (→"IE":string)
    n483 = feedback #5() -> (w114:u64)  [unwired: 1 in]
    n484 = feedback #6() -> (w112:dbl)  [unwired: 1 in]
    n485 = feedback #7() -> (w110:bool)  [unwired: 1 in]
    n486 = mathscript code="if (gt(index, 50) && le(index, 55))\nout = true;\nelse\nout = false;\nend\n\nif (gt(index, 300) && le(index, 305))\nout2 = true;\nelse\nout2 = false;\nend\n\nif (trigger == true)\nflag1 = true;\nflag2 = true;\nend\n\nif (flag1 == true)\nrand1 = rand_1;\nrand2 = rand_2;\nflag1 = false;\nend\n\nif (gt(index, rand1) && le(index, rand1+50))\nout3 = true;\nelse\nout3 = false;\nend\n\nif (gt(index, rand2) && le(index, rand2+30))\nout4 = true;\nelse\nout4 = false;\nend"("index"=w120, "trigger"=w119, "rand_1"=w118, "rand_2"=w117, "flag1"=w110, "rand1"=w114, "rand2"=w112) -> ("out"=→"startSimu":bool, "out2"=→"flagTime1":bool, "flag1"=w111:bool, "out3"=→"flagTime2":bool, "rand1"=w115:u64, "rand2"=w113:dbl, "out4"=→"flagTime3":bool)  [unwired: 1 in, 1 out]
    n487 = feedback-in #5(w115) -> ()
    n488 = feedback-in #6(w113) -> ()
    n489 = feedback-in #7(w111) -> ()
    n490 = Bundle("vec_2"=w168, "vec_3"=w170) -> (→"graph5":cluster{"vec_2":dbl[], "vec_3":dbl[]})  [unwired: 1 in]
    n491 = Number To Decimal String(number=w158) -> (decimal integer string=w156:string)  [unwired: 1 in]
    n492 = case shown="True" w127 {
      tunnel: w126 -> [w385 _]
      tunnel: [w385 dbl[] [0.0, 0.0, 0.0, 0.0, 0.0] ("freqFiltered")] -> w125
      frame False {
      }
      frame True {
      }
    }
    n493 = Concatenate Strings("SpO2: ", "" ("string"), w156) -> (→"spo2":string)
    n494 = node-c288() -> ()  [unwired: 1 in, 1 out]
  }
  n495 = node-c288(w92) -> ()  [unwired: 1 out]
